vi "CreateAlertDialog.vi"(0 "reference in":refnum<class "LcWebView.lvclass">, 5 "Error In":errorcluster) -> (14 "reference out":refnum<class "LcWebView.lvclass">, 19 "Error Out":errorcluster)   [LabVIEW 2018, in "LcWebView.lvclass"]
uses:
  LcWebView.lvclass
panel:
  out "Loaded":bool
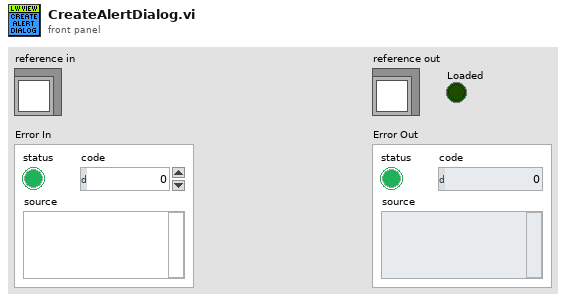
[diagram p1: front panel]
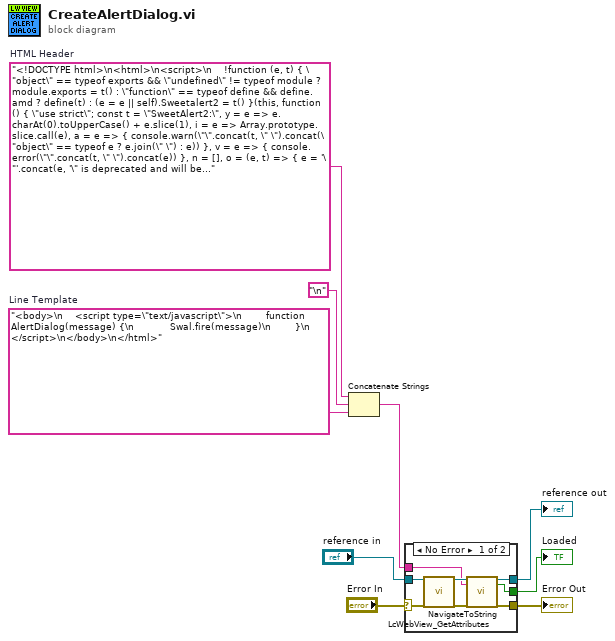
[diagram p0: block diagram]
diagram:
  w2 = "<body>\n    <script type=\"text/javascript\">\n        function AlertDialog(message) {\n            Swal.fire(message)\n        }\n    </script>\n</body>\n</html>"  # Line Template
  w4 = "<!DOCTYPE html>\n<html>\n<script>\n    !function (e, t) { \"object\" == typeof exports && \"undefined\" != typeof module ? module.exports = t() : \"function\" == typeof define && define.amd ? define(t) : (e = e || self).Sweetalert2 = t() }(this, function () { \"use strict\"; const t = \"SweetAlert2:\", y = e => e.charAt(0).toUpperCase() + e.slice(1), i = e => Array.prototype.slice.call(e), a = e => { console.warn(\"\".concat(t, \" \").concat(\"object\" == typeof e ? e.join(\" \") : e)) }, v = e => { console.error(\"\".concat(t, \" \").concat(e)) }, n = [], o = (e, t) => { e = '\"'.concat(e, '\" is deprecated and will be removed in the next major release. Please use \"').concat(t, '\" instead.'), n.includes(e) || (n.push(e), a(e)) }, w = e => \"function\" == typeof e ? e() : e, C = e => e && \"function\" == typeof e.toPromise, k = e => C(e) ? e.toPromise() : Promise.resolve(e), A = e => e && Promise.resolve(e) === e, r = { title: \"\", titleText: \"\", text: \"\", html: \"\", footer: \"\", icon: void 0, iconColor: void 0, iconHtml: void 0, template: void 0, toast: !1, showClass: { popup: \"swal2-show\", backdrop: \"swal2-backdrop-show\", icon: \"swal2-icon-show\" }, hideClass: { popup: \"swal2-hide\", backdrop: \"swal2-backdrop-hide\", icon: \"swal2-icon-hide\" }, customClass: {}, target: \"body\", color: void 0, backdrop: !0, heightAuto: !0, allowOutsideClick: !0, allowEscapeKey: !0, allowEnterKey: !0, stopKeydownPropagation: !0, keydownListenerCapture: !1, showConfirmButton: !0, showDenyButton: !1, showCancelButton: !1, preConfirm: void 0, preDeny: void 0, confirmButtonText: \"OK\", confirmButtonAriaLabel: \"\", confirmButtonColor: void 0, denyButtonText: \"No\", denyButtonAriaLabel: \"\", denyButtonColor: void 0, cancelButtonText: \"Cancel\", cancelButtonAriaLabel: \"\", cancelButtonColor: void 0, buttonsStyling: !0, reverseButtons: !1, focusConfirm: !0, focusDeny: !1, focusCancel: !1, returnFocus: !0, showCloseButton: !1, closeButtonHtml: \"&times;\", closeButtonAriaLabel: \"Close this dialog\", loaderHtml: \"\", showLoaderOnConfirm: !1, showLoaderOnDeny: !1, imageUrl: void 0, imageWidth: void 0, imageHeight: void 0, imageAlt: \"\", timer: void 0, timerProgressBar: !1, width: void 0, padding: void 0, background: void 0, input: void 0, inputPlaceholder: \"\", inputLabel: \"\", inputValue: \"\", inputOptions: {}, inputAutoTrim: !0, inputAttributes: {}, inputValidator: void 0, returnInputValueOnDeny: !1, validationMessage: void 0, grow: !1, position: \"center\", progressSteps: [], currentProgressStep: void 0, progressStepsDistance: void 0, willOpen: void 0, didOpen: void 0, didRender: void 0, willClose: void 0, didClose: void 0, didDestroy: void 0, scrollbarPadding: !0 }, s = [\"allowEscapeKey\", \"allowOutsideClick\", \"background\", \"buttonsStyling\", \"cancelButtonAriaLabel\", \"cancelButtonColor\", \"cancelButtonText\", \"closeButtonAriaLabel\", \"closeButtonHtml\", \"color\", \"confirmButtonAriaLabel\", \"confirmButtonColor\", \"confirmButtonText\", \"currentProgressStep\", \"customClass\", \"denyButtonAriaLabel\", \"denyButtonColor\", \"denyButtonText\", \"didClose\", \"didDestroy\", \"footer\", \"hideClass\", \"html\", \"icon\", \"iconColor\", \"iconHtml\", \"imageAlt\", \"imageHeight\", \"imageUrl\", \"imageWidth\", \"preConfirm\", \"preDeny\", \"progressSteps\", \"returnFocus\", \"reverseButtons\", \"showCancelButton\", \"showCloseButton\", \"showConfirmButton\", \"showDenyButton\", \"text\", \"title\", \"titleText\", \"willClose\"], c = {}, P = [\"allowOutsideClick\", \"allowEnterKey\", \"backdrop\", \"focusConfirm\", \"focusDeny\", \"focusCancel\", \"returnFocus\", \"heightAuto\", \"keydownListenerCapture\"], B = e => Object.prototype.hasOwnProperty.call(r, e), x = e => -1 !== s.indexOf(e), E = e => c[e], T = e => { !e.backdrop && e.allowOutsideClick && a('\"allowOutsideClick\" parameter requires `backdrop` parameter to be set to `true`'); for (const n in e) t = n, B(t) || a('Unknown parameter \"'.concat(t, '\"')), e.toast && (t = n, P.includes(t) && a('The parameter \"'.concat(t, '\" is incompatible with toasts'))), t = n, E(t) && o(t, E(t)); var t }; var e = e => { const t = {}; for (const n in e) t[e[n]] = \"swal2-\" + e[n]; return t }; const p = e([\"container\", \"shown\", \"height-auto\", \"iosfix\", \"popup\", \"modal\", \"no-backdrop\", \"no-transition\", \"toast\", \"toast-shown\", \"show\", \"hide\", \"close\", \"title\", \"html-container\", \"actions\", \"confirm\", \"deny\", \"cancel\", \"default-outline\", \"footer\", \"icon\", \"icon-content\", \"image\", \"input\", \"file\", \"range\", \"select\", \"radio\", \"checkbox\", \"label\", \"textarea\", \"inputerror\", \"input-label\", \"validation-message\", \"progress-steps\", \"active-progress-step\", \"progress-step\", \"progress-step-line\", \"loader\", \"loading\", \"styled\", \"top\", \"top-start\", \"top-end\", \"top-left\", \"top-right\", \"center\", \"center-start\", \"center-end\", \"center-left\", \"center-right\", \"bottom\", \"bottom-start\", \"bottom-end\", \"bottom-left\", \"bottom-right\", \"grow-row\", \"grow-column\", \"grow-fullscreen\", \"rtl\", \"timer-progress-bar\", \"timer-progress-bar-container\", \"scrollbar-measure\", \"icon-success\", \"icon-warning\", \"icon-info\", \"icon-question\", \"icon-error\"]), S = e([\"success\", \"warning\", \"info\", \"question\", \"error\"]), m = () => document.body.querySelector(\".\".concat(p.container)), L = e => { const t = m(); return t ? t.querySelector(e) : null }, O = e => L(\".\".concat(e)), g = () => O(p.popup), j = () => O(p.icon), M = () => O(p.title), D = () => O(p[\"html-container\"]), I = () => O(p.image), H = () => O(p[\"progress-steps\"]), q = () => O(p[\"validation-message\"]), V = () => L(\".\".concat(p.actions, \" .\").concat(p.confirm)), N = () => L(\".\".concat(p.actions, \" .\").concat(p.deny)); const R = () => L(\".\".concat(p.loader)), F = () => L(\".\".concat(p.actions, \" .\").concat(p.cancel)), U = () => O(p.actions), W = () => O(p.footer), z = () => O(p[\"timer-progress-bar\"]), _ = () => O(p.close), K = () => { const e = i(g().querySelectorAll('[tabindex]:not([tabindex=\"-1\"]):not([tabindex=\"0\"])')).sort((e, t) => { e = parseInt(e.getAttribute(\"tabindex\")), t = parseInt(t.getAttribute(\"tabindex\")); return t < e ? 1 : e < t ? -1 : 0 }); var t = i(g().querySelectorAll('\\n  a[href],\\n  area[href],\\n  input:not([disabled]),\\n  select:not([disabled]),\\n  textarea:not([disabled]),\\n  button:not([disabled]),\\n  iframe,\\n  object,\\n  embed,\\n  [tabindex=\"0\"],\\n  [contenteditable],\\n  audio[controls],\\n  video[controls],\\n  summary\\n')).filter(e => \"-1\" !== e.getAttribute(\"tabindex\")); return (t => { const n = []; for (let e = 0; e < t.length; e++)-1 === n.indexOf(t[e]) && n.push(t[e]); return n })(e.concat(t)).filter(e => ce(e)) }, Y = () => !$(document.body, p[\"toast-shown\"]) && !$(document.body, p[\"no-backdrop\"]), Z = () => g() && $(g(), p.toast); function J(e) { var t = 1 < arguments.length && void 0 !== arguments[1] && arguments[1]; const n = z(); ce(n) && (t && (n.style.transition = \"none\", n.style.width = \"100%\"), setTimeout(() => { n.style.transition = \"width \".concat(e / 1e3, \"s linear\"), n.style.width = \"0%\" }, 10)) } const X = { previousBodyPadding: null }, l = (t, e) => { if (t.textContent = \"\", e) { const n = new DOMParser, o = n.parseFromString(e, \"text/html\"); i(o.querySelector(\"head\").childNodes).forEach(e => { t.appendChild(e) }), i(o.querySelector(\"body\").childNodes).forEach(e => { t.appendChild(e) }) } }, $ = (t, e) => { if (!e) return !1; var n = e.split(/\\s+/); for (let e = 0; e < n.length; e++)if (!t.classList.contains(n[e])) return !1; return !0 }, G = (t, n) => { i(t.classList).forEach(e => { Object.values(p).includes(e) || Object.values(S).includes(e) || Object.values(n.showClass).includes(e) || t.classList.remove(e) }) }, Q = (e, t, n) => { if (G(e, t), t.customClass && t.customClass[n]) { if (\"string\" != typeof t.customClass[n] && !t.customClass[n].forEach) return a(\"Invalid type of customClass.\".concat(n, '! Expected string or iterable object, got \"').concat(typeof t.customClass[n], '\"')); u(e, t.customClass[n]) } }, ee = (e, t) => { if (!t) return null; switch (t) { case \"select\": case \"textarea\": case \"file\": return e.querySelector(\".\".concat(p.popup, \" > .\").concat(p[t])); case \"checkbox\": return e.querySelector(\".\".concat(p.popup, \" > .\").concat(p.checkbox, \" input\")); case \"radio\": return e.querySelector(\".\".concat(p.popup, \" > .\").concat(p.radio, \" input:checked\")) || e.querySelector(\".\".concat(p.popup, \" > .\").concat(p.radio, \" input:first-child\")); case \"range\": return e.querySelector(\".\".concat(p.popup, \" > .\").concat(p.range, \" input\")); default: return e.querySelector(\".\".concat(p.popup, \" > .\").concat(p.input)) } }, te = e => { var t; e.focus(), \"file\" !== e.type && (t = e.value, e.value = \"\", e.value = t) }, ne = (e, t, n) => { e && t && (t = \"string\" == typeof t ? t.split(/\\s+/).filter(Boolean) : t).forEach(t => { Array.isArray(e) ? e.forEach(e => { n ? e.classList.add(t) : e.classList.remove(t) }) : n ? e.classList.add(t) : e.classList.remove(t) }) }, u = (e, t) => { ne(e, t, !0) }, oe = (e, t) => { ne(e, t, !1) }, ie = (e, t) => { var n = i(e.childNodes); for (let e = 0; e < n.length; e++)if ($(n[e], t)) return n[e] }, ae = (e, t, n) => { (n = n === \"\".concat(parseInt(n)) ? parseInt(n) : n) || 0 === parseInt(n) ? e.style[t] = \"number\" == typeof n ? \"\".concat(n, \"px\") : n : e.style.removeProperty(t) }, d = function (e) { e.style.display = 1 < arguments.length && void 0 !== arguments[1] ? arguments[1] : \"flex\" }, h = e => { e.style.display = \"none\" }, re = (e, t, n, o) => { const i = e.querySelector(t); i && (i.style[n] = o) }, se = (e, t, n) => { t ? d(e, n) : h(e) }, ce = e => !(!e || !(e.offsetWidth || e.offsetHeight || e.getClientRects().length)), le = () => !ce(V()) && !ce(N()) && !ce(F()), ue = e => !!(e.scrollHeight > e.clientHeight), de = e => { const t = window.getComputedStyle(e); var e = parseFloat(t.getPropertyValue(\"animation-duration\") || \"0\"), n = parseFloat(t.getPropertyValue(\"transition-duration\") || \"0\"); return 0 < e || 0 < n }, pe = () => \"undefined\" == typeof window || \"undefined\" == typeof document, me = 100, f = {}, ge = () => { f.previousActiveElement && f.previousActiveElement.focus ? (f.previousActiveElement.focus(), f.previousActiveElement = null) : document.body && document.body.focus() }, he = o => new Promise(e => { if (!o) return e(); var t = window.scrollX, n = window.scrollY; f.restoreFocusTimeout = setTimeout(() => { ge(), e() }, me), window.scrollTo(t, n) }), fe = '\\n <div aria-labelledby=\"'.concat(p.title, '\" aria-describedby=\"').concat(p[\"html-container\"], '\" class=\"').concat(p.popup, '\" tabindex=\"-1\">\\n   <button type=\"button\" class=\"').concat(p.close, '\"></button>\\n   <ul class=\"').concat(p[\"progress-steps\"], '\"></ul>\\n   <div class=\"').concat(p.icon, '\"></div>\\n   <img class=\"').concat(p.image, '\" />\\n   <h2 class=\"').concat(p.title, '\" id=\"').concat(p.title, '\"></h2>\\n   <div class=\"').concat(p[\"html-container\"], '\" id=\"').concat(p[\"html-container\"], '\"></div>\\n   <input class=\"').concat(p.input, '\" />\\n   <input type=\"file\" class=\"').concat(p.file, '\" />\\n   <div class=\"').concat(p.range, '\">\\n     <input type=\"range\" />\\n     <output></output>\\n   </div>\\n   <select class=\"').concat(p.select, '\"></select>\\n   <div class=\"').concat(p.radio, '\"></div>\\n   <label for=\"').concat(p.checkbox, '\" class=\"').concat(p.checkbox, '\">\\n     <input type=\"checkbox\" />\\n     <span class=\"').concat(p.label, '\"></span>\\n   </label>\\n   <textarea class=\"').concat(p.textarea, '\"></textarea>\\n   <div class=\"').concat(p[\"validation-message\"], '\" id=\"').concat(p[\"validation-message\"], '\"></div>\\n   <div class=\"').concat(p.actions, '\">\\n     <div class=\"').concat(p.loader, '\"></div>\\n     <button type=\"button\" class=\"').concat(p.confirm, '\"></button>\\n     <button type=\"button\" class=\"').concat(p.deny, '\"></button>\\n     <button type=\"button\" class=\"').concat(p.cancel, '\"></button>\\n   </div>\\n   <div class=\"').concat(p.footer, '\"></div>\\n   <div class=\"').concat(p[\"timer-progress-bar-container\"], '\">\\n     <div class=\"').concat(p[\"timer-progress-bar\"], '\"></div>\\n   </div>\\n </div>\\n').replace(/(^|\\n)\\s*/g, \"\"), be = () => { const e = m(); return !!e && (e.remove(), oe([document.documentElement, document.body], [p[\"no-backdrop\"], p[\"toast-shown\"], p[\"has-column\"]]), !0) }, ye = () => { f.currentInstance.resetValidationMessage() }, ve = () => { const e = g(), t = ie(e, p.input), n = ie(e, p.file), o = e.querySelector(\".\".concat(p.range, \" input\")), i = e.querySelector(\".\".concat(p.range, \" output\")), a = ie(e, p.select), r = e.querySelector(\".\".concat(p.checkbox, \" input\")), s = ie(e, p.textarea); t.oninput = ye, n.onchange = ye, a.onchange = ye, r.onchange = ye, s.oninput = ye, o.oninput = () => { ye(), i.value = o.value }, o.onchange = () => { ye(), o.nextSibling.value = o.value } }, we = e => \"string\" == typeof e ? document.querySelector(e) : e, Ce = e => { const t = g(); t.setAttribute(\"role\", e.toast ? \"alert\" : \"dialog\"), t.setAttribute(\"aria-live\", e.toast ? \"polite\" : \"assertive\"), e.toast || t.setAttribute(\"aria-modal\", \"true\") }, ke = e => { \"rtl\" === window.getComputedStyle(e).direction && u(m(), p.rtl) }, Ae = (e, t) => { if (e instanceof HTMLElement) t.appendChild(e); else if (\"object\" == typeof e) { var n = e, o = t; if (n.jquery) Pe(o, n); else l(o, n.toString()) } else e && l(t, e) }, Pe = (t, n) => { if (t.textContent = \"\", 0 in n) for (let e = 0; e in n; e++)t.appendChild(n[e].cloneNode(!0)); else t.appendChild(n.cloneNode(!0)) }, Be = (() => { if (pe()) return !1; var e = document.createElement(\"div\"), t = { WebkitAnimation: \"webkitAnimationEnd\", animation: \"animationend\" }; for (const n in t) if (Object.prototype.hasOwnProperty.call(t, n) && void 0 !== e.style[n]) return t[n]; return !1 })(), xe = (e, t) => { var n, o, i, a, r, s = U(), c = R(); (t.showConfirmButton || t.showDenyButton || t.showCancelButton ? d : h)(s), Q(s, t, \"actions\"), s = s, n = c, o = t, i = V(), a = N(), r = F(), Ee(i, \"confirm\", o), Ee(a, \"deny\", o), Ee(r, \"cancel\", o), function (e, t, n, o) { if (!o.buttonsStyling) return oe([e, t, n], p.styled); u([e, t, n], p.styled), o.confirmButtonColor && (e.style.backgroundColor = o.confirmButtonColor, u(e, p[\"default-outline\"])); o.denyButtonColor && (t.style.backgroundColor = o.denyButtonColor, u(t, p[\"default-outline\"])); o.cancelButtonColor && (n.style.backgroundColor = o.cancelButtonColor, u(n, p[\"default-outline\"])) }(i, a, r, o), o.reverseButtons && (o.toast ? (s.insertBefore(r, i), s.insertBefore(a, i)) : (s.insertBefore(r, n), s.insertBefore(a, n), s.insertBefore(i, n))), l(c, t.loaderHtml), Q(c, t, \"loader\") }; function Ee(e, t, n) { se(e, n[\"show\".concat(y(t), \"Button\")], \"inline-block\"), l(e, n[\"\".concat(t, \"ButtonText\")]), e.setAttribute(\"aria-label\", n[\"\".concat(t, \"ButtonAriaLabel\")]), e.className = p[t], Q(e, n, \"\".concat(t, \"Button\")), u(e, n[\"\".concat(t, \"ButtonClass\")]) } const Te = (e, t) => { var n, o, i = m(); i && (o = i, \"string\" == typeof (n = t.backdrop) ? o.style.background = n : n || u([document.documentElement, document.body], p[\"no-backdrop\"]), o = i, (n = t.position) in p ? u(o, p[n]) : (a('The \"position\" parameter is not valid, defaulting to \"center\"'), u(o, p.center)), n = i, !(o = t.grow) || \"string\" != typeof o || (o = \"grow-\".concat(o)) in p && u(n, p[o]), Q(i, t, \"container\")) }; var b = { awaitingPromise: new WeakMap, promise: new WeakMap, innerParams: new WeakMap, domCache: new WeakMap }; const Se = [\"input\", \"file\", \"range\", \"select\", \"radio\", \"checkbox\", \"textarea\"], Le = (e, r) => { const s = g(); var t, e = b.innerParams.get(e); const c = !e || r.input !== e.input; Se.forEach(e => { var t = p[e]; const n = ie(s, t); { var o = r.inputAttributes; const i = ee(g(), e); if (i) { Oe(i); for (const a in o) i.setAttribute(a, o[a]) } } n.className = t, c && h(n) }), r.input && (c && (e => { if (!Ie[e.input]) return v('Unexpected type of input! Expected \"text\", \"email\", \"password\", \"number\", \"tel\", \"select\", \"radio\", \"checkbox\", \"textarea\", \"file\" or \"url\", got \"'.concat(e.input, '\"')); const t = De(e.input), n = Ie[e.input](t, e); d(n), setTimeout(() => { te(n) }) })(r), e = r, t = De(e.input), e.customClass && u(t, e.customClass.input)) }, Oe = t => { for (let e = 0; e < t.attributes.length; e++) { var n = t.attributes[e].name;[\"type\", \"value\", \"style\"].includes(n) || t.removeAttribute(n) } }, je = (e, t) => { e.placeholder && !t.inputPlaceholder || (e.placeholder = t.inputPlaceholder) }, Me = (e, t, n) => { if (n.inputLabel) { e.id = p.input; const i = document.createElement(\"label\"); var o = p[\"input-label\"]; i.setAttribute(\"for\", e.id), i.className = o, u(i, n.customClass.inputLabel), i.innerText = n.inputLabel, t.insertAdjacentElement(\"beforebegin\", i) } }, De = e => { e = p[e] || p.input; return ie(g(), e) }, Ie = {}, He = (Ie.text = Ie.email = Ie.password = Ie.number = Ie.tel = Ie.url = (e, t) => (\"string\" == typeof t.inputValue || \"number\" == typeof t.inputValue ? e.value = t.inputValue : A(t.inputValue) || a('Unexpected type of inputValue! Expected \"string\", \"number\" or \"Promise\", got \"'.concat(typeof t.inputValue, '\"')), Me(e, e, t), je(e, t), e.type = t.input, e), Ie.file = (e, t) => (Me(e, e, t), je(e, t), e), Ie.range = (e, t) => { const n = e.querySelector(\"input\"), o = e.querySelector(\"output\"); return n.value = t.inputValue, n.type = t.input, o.value = t.inputValue, Me(n, e, t), e }, Ie.select = (e, t) => { if (e.textContent = \"\", t.inputPlaceholder) { const n = document.createElement(\"option\"); l(n, t.inputPlaceholder), n.value = \"\", n.disabled = !0, n.selected = !0, e.appendChild(n) } return Me(e, e, t), e }, Ie.radio = e => (e.textContent = \"\", e), Ie.checkbox = (e, t) => { const n = ee(g(), \"checkbox\"); n.value = \"1\", n.id = p.checkbox, n.checked = Boolean(t.inputValue); var o = e.querySelector(\"span\"); return l(o, t.inputPlaceholder), e }, Ie.textarea = (n, e) => { n.value = e.inputValue, je(n, e), Me(n, n, e); return setTimeout(() => { if (\"MutationObserver\" in window) { const t = parseInt(window.getComputedStyle(g()).width); new MutationObserver(() => { var e = n.offsetWidth + (e = n, parseInt(window.getComputedStyle(e).marginLeft) + parseInt(window.getComputedStyle(e).marginRight)); e > t ? g().style.width = \"\".concat(e, \"px\") : g().style.width = null }).observe(n, { attributes: !0, attributeFilter: [\"style\"] }) } }), n }, (e, t) => { const n = D(); Q(n, t, \"htmlContainer\"), t.html ? (Ae(t.html, n), d(n, \"block\")) : t.text ? (n.textContent = t.text, d(n, \"block\")) : h(n), Le(e, t) }), qe = (e, t) => { var n = W(); se(n, t.footer), t.footer && Ae(t.footer, n), Q(n, t, \"footer\") }, Ve = (e, t) => { const n = _(); l(n, t.closeButtonHtml), Q(n, t, \"closeButton\"), se(n, t.showCloseButton), n.setAttribute(\"aria-label\", t.closeButtonAriaLabel) }, Ne = (e, t) => { var e = b.innerParams.get(e), n = j(); return e && t.icon === e.icon ? (ze(n, t), void Re(n, t)) : t.icon || t.iconHtml ? t.icon && -1 === Object.keys(S).indexOf(t.icon) ? (v('Unknown icon! Expected \"success\", \"error\", \"warning\", \"info\" or \"question\", got \"'.concat(t.icon, '\"')), h(n)) : (d(n), ze(n, t), Re(n, t), void u(n, t.showClass.icon)) : h(n) }, Re = (e, t) => { for (const n in S) t.icon !== n && oe(e, S[n]); u(e, S[t.icon]), _e(e, t), Fe(), Q(e, t, \"icon\") }, Fe = () => { const e = g(); var t = window.getComputedStyle(e).getPropertyValue(\"background-color\"); const n = e.querySelectorAll(\"[class^=swal2-success-circular-line], .swal2-success-fix\"); for (let e = 0; e < n.length; e++)n[e].style.backgroundColor = t }, Ue = '\\n  <div class=\"swal2-success-circular-line-left\"></div>\\n  <span class=\"swal2-success-line-tip\"></span> <span class=\"swal2-success-line-long\"></span>\\n  <div class=\"swal2-success-ring\"></div> <div class=\"swal2-success-fix\"></div>\\n  <div class=\"swal2-success-circular-line-right\"></div>\\n', We = '\\n  <span class=\"swal2-x-mark\">\\n    <span class=\"swal2-x-mark-line-left\"></span>\\n    <span class=\"swal2-x-mark-line-right\"></span>\\n  </span>\\n', ze = (e, t) => { var n; e.textContent = \"\", t.iconHtml ? l(e, Ke(t.iconHtml)) : \"success\" === t.icon ? l(e, Ue) : \"error\" === t.icon ? l(e, We) : (n = { question: \"?\", warning: \"!\", info: \"i\" }, l(e, Ke(n[t.icon]))) }, _e = (e, t) => { if (t.iconColor) { e.style.color = t.iconColor, e.style.borderColor = t.iconColor; for (const n of [\".swal2-success-line-tip\", \".swal2-success-line-long\", \".swal2-x-mark-line-left\", \".swal2-x-mark-line-right\"]) re(e, n, \"backgroundColor\", t.iconColor); re(e, \".swal2-success-ring\", \"borderColor\", t.iconColor) } }, Ke = e => '<div class=\"'.concat(p[\"icon-content\"], '\">').concat(e, \"</div>\"), Ye = (e, t) => { const n = I(); if (!t.imageUrl) return h(n); d(n, \"\"), n.setAttribute(\"src\", t.imageUrl), n.setAttribute(\"alt\", t.imageAlt), ae(n, \"width\", t.imageWidth), ae(n, \"height\", t.imageHeight), n.className = p.image, Q(n, t, \"image\") }, Ze = (e, o) => { const i = H(); if (!o.progressSteps || 0 === o.progressSteps.length) return h(i); d(i), i.textContent = \"\", o.currentProgressStep >= o.progressSteps.length && a(\"Invalid currentProgressStep parameter, it should be less than progressSteps.length (currentProgressStep like JS arrays starts from 0)\"), o.progressSteps.forEach((e, t) => { e = e, n = document.createElement(\"li\"), u(n, p[\"progress-step\"]), l(n, e); var n, e = n; i.appendChild(e), t === o.currentProgressStep && u(e, p[\"active-progress-step\"]), t !== o.progressSteps.length - 1 && (n = (e => { const t = document.createElement(\"li\"); return u(t, p[\"progress-step-line\"]), e.progressStepsDistance && (t.style.width = e.progressStepsDistance), t })(o), i.appendChild(n)) }) }, Je = (e, t) => { const n = M(); se(n, t.title || t.titleText, \"block\"), t.title && Ae(t.title, n), t.titleText && (n.innerText = t.titleText), Q(n, t, \"title\") }, Xe = (e, t) => { var n = m(); const o = g(); t.toast ? (ae(n, \"width\", t.width), o.style.width = \"100%\", o.insertBefore(R(), j())) : ae(o, \"width\", t.width), ae(o, \"padding\", t.padding), t.color && (o.style.color = t.color), t.background && (o.style.background = t.background), h(q()); n = o; (n.className = \"\".concat(p.popup, \" \").concat(ce(n) ? t.showClass.popup : \"\"), t.toast) ? (u([document.documentElement, document.body], p[\"toast-shown\"]), u(n, p.toast)) : u(n, p.modal); Q(n, t, \"popup\"), \"string\" == typeof t.customClass && u(n, t.customClass); t.icon && u(n, p[\"icon-\".concat(t.icon)]) }, $e = (e, t) => { Xe(e, t), Te(e, t), Ze(e, t), Ne(e, t), Ye(e, t), Je(e, t), Ve(e, t), He(e, t), xe(e, t), qe(e, t), \"function\" == typeof t.didRender && t.didRender(g()) }, Ge = Object.freeze({ cancel: \"cancel\", backdrop: \"backdrop\", close: \"close\", esc: \"esc\", timer: \"timer\" }), Qe = () => { const e = i(document.body.children); e.forEach(e => { e === m() || e.contains(m()) || (e.hasAttribute(\"aria-hidden\") && e.setAttribute(\"data-previous-aria-hidden\", e.getAttribute(\"aria-hidden\")), e.setAttribute(\"aria-hidden\", \"true\")) }) }, et = () => { const e = i(document.body.children); e.forEach(e => { e.hasAttribute(\"data-previous-aria-hidden\") ? (e.setAttribute(\"aria-hidden\", e.getAttribute(\"data-previous-aria-hidden\")), e.removeAttribute(\"data-previous-aria-hidden\")) : e.removeAttribute(\"aria-hidden\") }) }, tt = [\"swal-title\", \"swal-html\", \"swal-footer\"], nt = e => { const n = {}; return i(e.querySelectorAll(\"swal-param\")).forEach(e => { lt(e, [\"name\", \"value\"]); var t = e.getAttribute(\"name\"), e = e.getAttribute(\"value\"); \"boolean\" == typeof r[t] && \"false\" === e && (n[t] = !1), \"object\" == typeof r[t] && (n[t] = JSON.parse(e)) }), n }, ot = e => { const n = {}; return i(e.querySelectorAll(\"swal-button\")).forEach(e => { lt(e, [\"type\", \"color\", \"aria-label\"]); var t = e.getAttribute(\"type\"); n[\"\".concat(t, \"ButtonText\")] = e.innerHTML, n[\"show\".concat(y(t), \"Button\")] = !0, e.hasAttribute(\"color\") && (n[\"\".concat(t, \"ButtonColor\")] = e.getAttribute(\"color\")), e.hasAttribute(\"aria-label\") && (n[\"\".concat(t, \"ButtonAriaLabel\")] = e.getAttribute(\"aria-label\")) }), n }, it = e => { const t = {}, n = e.querySelector(\"swal-image\"); return n && (lt(n, [\"src\", \"width\", \"height\", \"alt\"]), n.hasAttribute(\"src\") && (t.imageUrl = n.getAttribute(\"src\")), n.hasAttribute(\"width\") && (t.imageWidth = n.getAttribute(\"width\")), n.hasAttribute(\"height\") && (t.imageHeight = n.getAttribute(\"height\")), n.hasAttribute(\"alt\") && (t.imageAlt = n.getAttribute(\"alt\"))), t }, at = e => { const t = {}, n = e.querySelector(\"swal-icon\"); return n && (lt(n, [\"type\", \"color\"]), n.hasAttribute(\"type\") && (t.icon = n.getAttribute(\"type\")), n.hasAttribute(\"color\") && (t.iconColor = n.getAttribute(\"color\")), t.iconHtml = n.innerHTML), t }, rt = e => { const n = {}, t = e.querySelector(\"swal-input\"); t && (lt(t, [\"type\", \"label\", \"placeholder\", \"value\"]), n.input = t.getAttribute(\"type\") || \"text\", t.hasAttribute(\"label\") && (n.inputLabel = t.getAttribute(\"label\")), t.hasAttribute(\"placeholder\") && (n.inputPlaceholder = t.getAttribute(\"placeholder\")), t.hasAttribute(\"value\") && (n.inputValue = t.getAttribute(\"value\"))); e = e.querySelectorAll(\"swal-input-option\"); return e.length && (n.inputOptions = {}, i(e).forEach(e => { lt(e, [\"value\"]); var t = e.getAttribute(\"value\"), e = e.innerHTML; n.inputOptions[t] = e })), n }, st = (e, t) => { const n = {}; for (const o in t) { const i = t[o], a = e.querySelector(i); a && (lt(a, []), n[i.replace(/^swal-/, \"\")] = a.innerHTML.trim()) } return n }, ct = e => { const t = tt.concat([\"swal-param\", \"swal-button\", \"swal-image\", \"swal-icon\", \"swal-input\", \"swal-input-option\"]); i(e.children).forEach(e => { e = e.tagName.toLowerCase(); -1 === t.indexOf(e) && a(\"Unrecognized element <\".concat(e, \">\")) }) }, lt = (t, n) => { i(t.attributes).forEach(e => { -1 === n.indexOf(e.name) && a(['Unrecognized attribute \"'.concat(e.name, '\" on <').concat(t.tagName.toLowerCase(), \">.\"), \"\".concat(n.length ? \"Allowed attributes are: \".concat(n.join(\", \")) : \"To set the value, use HTML within the element.\")]) }) }; var ut = { email: (e, t) => /^[a-zA-Z0-9.+_-]+@[a-zA-Z0-9.-]+\\.[a-zA-Z0-9-]{2,24}$/.test(e) ? Promise.resolve() : Promise.resolve(t || \"Invalid email address\"), url: (e, t) => /^https?:\\/\\/(www\\.)?[-a-zA-Z0-9@:%._+~#=]{1,256}\\.[a-z]{2,63}\\b([-a-zA-Z0-9@:%_+.~#?&/=]*)$/.test(e) ? Promise.resolve() : Promise.resolve(t || \"Invalid URL\") }; function dt(e) { (t = e).inputValidator || Object.keys(ut).forEach(e => { t.input === e && (t.inputValidator = ut[e]) }), e.showLoaderOnConfirm && !e.preConfirm && a(\"showLoaderOnConfirm is set to true, but preConfirm is not defined.\\nshowLoaderOnConfirm should be used together with preConfirm, see usage example:\\nhttps://sweetalert2.github.io/#ajax-request\"), (n = e).target && (\"string\" != typeof n.target || document.querySelector(n.target)) && (\"string\" == typeof n.target || n.target.appendChild) || (a('Target parameter is not valid, defaulting to \"body\"'), n.target = \"body\"), \"string\" == typeof e.title && (e.title = e.title.split(\"\\n\").join(\"<br />\")); var t, n = e, e = be(); if (pe()) v(\"SweetAlert2 requires document to initialize\"); else { const o = document.createElement(\"div\"), i = (o.className = p.container, e && u(o, p[\"no-transition\"]), l(o, fe), we(n.target)); i.appendChild(o), Ce(n), ke(i), ve() } } class pt { constructor(e, t) { this.callback = e, this.remaining = t, this.running = !1, this.start() } start() { return this.running || (this.running = !0, this.started = new Date, this.id = setTimeout(this.callback, this.remaining)), this.remaining } stop() { return this.running && (this.running = !1, clearTimeout(this.id), this.remaining -= (new Date).getTime() - this.started.getTime()), this.remaining } increase(e) { var t = this.running; return t && this.stop(), this.remaining += e, t && this.start(), this.remaining } getTimerLeft() { return this.running && (this.stop(), this.start()), this.remaining } isRunning() { return this.running } } const mt = () => { null === X.previousBodyPadding && document.body.scrollHeight > window.innerHeight && (X.previousBodyPadding = parseInt(window.getComputedStyle(document.body).getPropertyValue(\"padding-right\")), document.body.style.paddingRight = \"\".concat(X.previousBodyPadding + (() => { const e = document.createElement(\"div\"); e.className = p[\"scrollbar-measure\"], document.body.appendChild(e); var t = e.getBoundingClientRect().width - e.clientWidth; return document.body.removeChild(e), t })(), \"px\")) }, gt = () => { null !== X.previousBodyPadding && (document.body.style.paddingRight = \"\".concat(X.previousBodyPadding, \"px\"), X.previousBodyPadding = null) }, ht = () => { var e = /iPad|iPhone|iPod/.test(navigator.userAgent) && !window.MSStream || \"MacIntel\" === navigator.platform && 1 < navigator.maxTouchPoints; if (e && !$(document.body, p.iosfix)) { var t, e = document.body.scrollTop; document.body.style.top = \"\".concat(-1 * e, \"px\"), u(document.body, p.iosfix); { const n = m(); let t; n.ontouchstart = e => { t = ft(e) }, n.ontouchmove = e => { t && (e.preventDefault(), e.stopPropagation()) } } { const o = navigator.userAgent, i = !!o.match(/iPad/i) || !!o.match(/iPhone/i), a = !!o.match(/WebKit/i), r = i && a && !o.match(/CriOS/i); r && (t = 44, g().scrollHeight > window.innerHeight - 44 && (m().style.paddingBottom = \"\".concat(44, \"px\"))) } } }, ft = e => { var t, n = e.target, o = m(); return !((t = e).touches && t.touches.length && \"stylus\" === t.touches[0].touchType || (t = e).touches && 1 < t.touches.length) && (n === o || !(ue(o) || \"INPUT\" === n.tagName || \"TEXTAREA\" === n.tagName || ue(D()) && D().contains(n))) }, bt = () => { var e; $(document.body, p.iosfix) && (e = parseInt(document.body.style.top, 10), oe(document.body, p.iosfix), document.body.style.top = \"\", document.body.scrollTop = -1 * e) }, yt = 10, vt = e => { const t = g(); if (e.target === t) { const n = m(); t.removeEventListener(Be, vt), n.style.overflowY = \"auto\" } }, wt = (e, t) => { Be && de(t) ? (e.style.overflowY = \"hidden\", t.addEventListener(Be, vt)) : e.style.overflowY = \"auto\" }, Ct = (e, t, n) => { ht(), t && \"hidden\" !== n && mt(), setTimeout(() => { e.scrollTop = 0 }) }, kt = (e, t, n) => { u(e, n.showClass.backdrop), t.style.setProperty(\"opacity\", \"0\", \"important\"), d(t, \"grid\"), setTimeout(() => { u(t, n.showClass.popup), t.style.removeProperty(\"opacity\") }, yt), u([document.documentElement, document.body], p.shown), n.heightAuto && n.backdrop && !n.toast && u([document.documentElement, document.body], p[\"height-auto\"]) }, At = e => { let t = g(); t || new vn, t = g(); var n = R(); if (Z()) h(j()); else { var o = t; const i = U(), a = R(); !e && ce(V()) && (e = V()); d(i), e && (h(e), a.setAttribute(\"data-button-to-replace\", e.className)); a.parentNode.insertBefore(a, e), u([o, i], p.loading) } d(n), t.setAttribute(\"data-loading\", !0), t.setAttribute(\"aria-busy\", !0), t.focus() }, Pt = (t, n) => { const o = g(), i = e => xt[n.input](o, Et(e), n); C(n.inputOptions) || A(n.inputOptions) ? (At(V()), k(n.inputOptions).then(e => { t.hideLoading(), i(e) })) : \"object\" == typeof n.inputOptions ? i(n.inputOptions) : v(\"Unexpected type of inputOptions! Expected object, Map or Promise, got \".concat(typeof n.inputOptions)) }, Bt = (t, n) => { const o = t.getInput(); h(o), k(n.inputValue).then(e => { o.value = \"number\" === n.input ? parseFloat(e) || 0 : \"\".concat(e), d(o), o.focus(), t.hideLoading() }).catch(e => { v(\"Error in inputValue promise: \".concat(e)), o.value = \"\", d(o), o.focus(), t.hideLoading() }) }, xt = { select: (e, t, i) => { const a = ie(e, p.select), r = (e, t, n) => { const o = document.createElement(\"option\"); o.value = n, l(o, t), o.selected = Tt(n, i.inputValue), e.appendChild(o) }; t.forEach(e => { var t = e[0]; const n = e[1]; if (Array.isArray(n)) { const o = document.createElement(\"optgroup\"); o.label = t, o.disabled = !1, a.appendChild(o), n.forEach(e => r(o, e[1], e[0])) } else r(a, n, t) }), a.focus() }, radio: (e, t, a) => { const r = ie(e, p.radio), n = (t.forEach(e => { var t = e[0], e = e[1]; const n = document.createElement(\"input\"), o = document.createElement(\"label\"), i = (n.type = \"radio\", n.name = p.radio, n.value = t, Tt(t, a.inputValue) && (n.checked = !0), document.createElement(\"span\")); l(i, e), i.className = p.label, o.appendChild(n), o.appendChild(i), r.appendChild(o) }), r.querySelectorAll(\"input\")); n.length && n[0].focus() } }, Et = n => { const o = []; return \"undefined\" != typeof Map && n instanceof Map ? n.forEach((e, t) => { let n = e; \"object\" == typeof n && (n = Et(n)), o.push([t, n]) }) : Object.keys(n).forEach(e => { let t = n[e]; \"object\" == typeof t && (t = Et(t)), o.push([e, t]) }), o }, Tt = (e, t) => t && t.toString() === e.toString(), St = (e, t) => { var n = b.innerParams.get(e); if (!n.input) return v('The \"input\" parameter is needed to be set when using returnInputValueOn'.concat(y(t))); var o = ((e, t) => { const n = e.getInput(); if (!n) return null; switch (t.input) { case \"checkbox\": return n.checked ? 1 : 0; case \"radio\": return (o = n).checked ? o.value : null; case \"file\": return (o = n).files.length ? null !== o.getAttribute(\"multiple\") ? o.files : o.files[0] : null; default: return t.inputAutoTrim ? n.value.trim() : n.value }var o })(e, n); if (n.inputValidator) { var i = e; var a = o; var r = t; const s = b.innerParams.get(i), c = (i.disableInput(), Promise.resolve().then(() => k(s.inputValidator(a, s.validationMessage)))); c.then(e => { i.enableButtons(), i.enableInput(), e ? i.showValidationMessage(e) : (\"deny\" === r ? Lt : Mt)(i, a) }) } else e.getInput().checkValidity() ? (\"deny\" === t ? Lt : Mt)(e, o) : (e.enableButtons(), e.showValidationMessage(n.validationMessage)) }, Lt = (t, n) => { const e = b.innerParams.get(t || void 0); if (e.showLoaderOnDeny && At(N()), e.preDeny) { b.awaitingPromise.set(t || void 0, !0); const o = Promise.resolve().then(() => k(e.preDeny(n, e.validationMessage))); o.then(e => { !1 === e ? t.hideLoading() : t.closePopup({ isDenied: !0, value: void 0 === e ? n : e }) }).catch(e => jt(t || void 0, e)) } else t.closePopup({ isDenied: !0, value: n }) }, Ot = (e, t) => { e.closePopup({ isConfirmed: !0, value: t }) }, jt = (e, t) => { e.rejectPromise(t) }, Mt = (t, n) => { const e = b.innerParams.get(t || void 0); if (e.showLoaderOnConfirm && At(), e.preConfirm) { t.resetValidationMessage(), b.awaitingPromise.set(t || void 0, !0); const o = Promise.resolve().then(() => k(e.preConfirm(n, e.validationMessage))); o.then(e => { ce(q()) || !1 === e ? t.hideLoading() : Ot(t, void 0 === e ? n : e) }).catch(e => jt(t || void 0, e)) } else Ot(t, n) }, Dt = (n, e, o) => { e.popup.onclick = () => { var e, t = b.innerParams.get(n); t && ((e = t).showConfirmButton || e.showDenyButton || e.showCancelButton || e.showCloseButton || t.timer || t.input) || o(Ge.close) } }; let It = !1; const Ht = t => { t.popup.onmousedown = () => { t.container.onmouseup = function (e) { t.container.onmouseup = void 0, e.target === t.container && (It = !0) } } }, qt = t => { t.container.onmousedown = () => { t.popup.onmouseup = function (e) { t.popup.onmouseup = void 0, e.target !== t.popup && !t.popup.contains(e.target) || (It = !0) } } }, Vt = (n, o, i) => { o.container.onclick = e => { var t = b.innerParams.get(n); It ? It = !1 : e.target === o.container && w(t.allowOutsideClick) && i(Ge.backdrop) } }; const Nt = () => V() && V().click(); const Rt = (e, t, n) => { const o = K(); if (o.length) return (t += n) === o.length ? t = 0 : -1 === t && (t = o.length - 1), o[t].focus(); g().focus() }, Ft = [\"ArrowRight\", \"ArrowDown\"], Ut = [\"ArrowLeft\", \"ArrowUp\"], Wt = (e, n, o) => { var i = b.innerParams.get(e); if (i) if (i.stopKeydownPropagation && n.stopPropagation(), \"Enter\" === n.key) e = e, a = n, t = i, w(t.allowEnterKey) && !a.isComposing && a.target && e.getInput() && a.target.outerHTML === e.getInput().outerHTML && ([\"textarea\", \"file\"].includes(t.input) || (Nt(), a.preventDefault())); else if (\"Tab\" !== n.key) { if ([...Ft, ...Ut].includes(n.key)) { e = n.key; const s = V(), c = N(), d = F(); if ([s, c, d].includes(document.activeElement)) { var t = Ft.includes(e) ? \"nextElementSibling\" : \"previousElementSibling\"; const l = document.activeElement[t]; l instanceof HTMLElement && l.focus() } } else if (\"Escape\" === n.key) { var a = n, e = i; if (w(e.allowEscapeKey)) { a.preventDefault(); o(Ge.esc) } } } else { e = n; o = i; var u = e.target, r = K(); let t = -1; for (let e = 0; e < r.length; e++)if (u === r[e]) { t = e; break } e.shiftKey ? Rt(o, t, -1) : Rt(o, t, 1); e.stopPropagation(), e.preventDefault() } }, zt = e => \"object\" == typeof e && e.jquery, _t = e => e instanceof Element || zt(e); const Kt = () => { if (f.timeout) { { const n = z(); var e = parseInt(window.getComputedStyle(n).width), t = (n.style.removeProperty(\"transition\"), n.style.width = \"100%\", parseInt(window.getComputedStyle(n).width)), e = e / t * 100; n.style.removeProperty(\"transition\"), n.style.width = \"\".concat(e, \"%\") } return f.timeout.stop() } }, Yt = () => { var e; if (f.timeout) return e = f.timeout.start(), J(e), e }; let Zt = !1; const Jt = {}; const Xt = t => { for (let e = t.target; e && e !== document; e = e.parentNode)for (const o in Jt) { var n = e.getAttribute(o); if (n) return void Jt[o].fire({ template: n }) } }; e = Object.freeze({ isValidParameter: B, isUpdatableParameter: x, isDeprecatedParameter: E, argsToParams: n => { const o = {}; return \"object\" != typeof n[0] || _t(n[0]) ? [\"title\", \"html\", \"icon\"].forEach((e, t) => { t = n[t]; \"string\" == typeof t || _t(t) ? o[e] = t : void 0 !== t && v(\"Unexpected type of \".concat(e, '! Expected \"string\" or \"Element\", got ').concat(typeof t)) }) : Object.assign(o, n[0]), o }, isVisible: () => ce(g()), clickConfirm: Nt, clickDeny: () => N() && N().click(), clickCancel: () => F() && F().click(), getContainer: m, getPopup: g, getTitle: M, getHtmlContainer: D, getImage: I, getIcon: j, getInputLabel: () => O(p[\"input-label\"]), getCloseButton: _, getActions: U, getConfirmButton: V, getDenyButton: N, getCancelButton: F, getLoader: R, getFooter: W, getTimerProgressBar: z, getFocusableElements: K, getValidationMessage: q, isLoading: () => g().hasAttribute(\"data-loading\"), fire: function () { for (var e = arguments.length, t = new Array(e), n = 0; n < e; n++)t[n] = arguments[n]; return new this(...t) }, mixin: function (n) { class e extends this{ _main(e, t) { return super._main(e, Object.assign({}, n, t)) } } return e }, showLoading: At, enableLoading: At, getTimerLeft: () => f.timeout && f.timeout.getTimerLeft(), stopTimer: Kt, resumeTimer: Yt, toggleTimer: () => { var e = f.timeout; return e && (e.running ? Kt : Yt)() }, increaseTimer: e => { if (f.timeout) return e = f.timeout.increase(e), J(e, !0), e }, isTimerRunning: () => f.timeout && f.timeout.isRunning(), bindClickHandler: function () { var e = 0 < arguments.length && void 0 !== arguments[0] ? arguments[0] : \"data-swal-template\"; Jt[e] = this, Zt || (document.body.addEventListener(\"click\", Xt), Zt = !0) } }); function $t() { var e, t = b.innerParams.get(this); if (t) { const n = b.domCache.get(this); h(n.loader), Z() ? t.icon && d(j()) : (t = n, (e = t.popup.getElementsByClassName(t.loader.getAttribute(\"data-button-to-replace\"))).length ? d(e[0], \"inline-block\") : le() && h(t.actions)), oe([n.popup, n.actions], p.loading), n.popup.removeAttribute(\"aria-busy\"), n.popup.removeAttribute(\"data-loading\"), n.confirmButton.disabled = !1, n.denyButton.disabled = !1, n.cancelButton.disabled = !1 } } var Gt = { swalPromiseResolve: new WeakMap, swalPromiseReject: new WeakMap }; function Qt(e, t, n, o) { Z() ? on(e, o) : (he(n).then(() => on(e, o)), f.keydownTarget.removeEventListener(\"keydown\", f.keydownHandler, { capture: f.keydownListenerCapture }), f.keydownHandlerAdded = !1), /^((?!chrome|android).)*safari/i.test(navigator.userAgent) ? (t.setAttribute(\"style\", \"display:none !important\"), t.removeAttribute(\"class\"), t.innerHTML = \"\") : t.remove(), Y() && (gt(), bt(), et()), oe([document.documentElement, document.body], [p.shown, p[\"height-auto\"], p[\"no-backdrop\"], p[\"toast-shown\"]]) } function en(e) { e = void 0 !== (n = e) ? Object.assign({ isConfirmed: !1, isDenied: !1, isDismissed: !1 }, n) : { isConfirmed: !1, isDenied: !1, isDismissed: !0 }; const t = Gt.swalPromiseResolve.get(this); var n = (e => { const t = g(); if (!t) return false; const n = b.innerParams.get(e); if (!n || $(t, n.hideClass.popup)) return false; oe(t, n.showClass.popup), u(t, n.hideClass.popup); const o = m(); return oe(o, n.showClass.backdrop), u(o, n.hideClass.backdrop), nn(e, t, n), true })(this); this.isAwaitingPromise() ? e.isDismissed || (tn(this), t(e)) : n && t(e) } const tn = e => { e.isAwaitingPromise() && (b.awaitingPromise.delete(e), b.innerParams.get(e) || e._destroy()) }, nn = (e, t, n) => { var o, i, a, r = m(), s = Be && de(t); \"function\" == typeof n.willClose && n.willClose(t), s ? (s = e, o = t, t = r, i = n.returnFocus, a = n.didClose, f.swalCloseEventFinishedCallback = Qt.bind(null, s, t, i, a), o.addEventListener(Be, function (e) { e.target === o && (f.swalCloseEventFinishedCallback(), delete f.swalCloseEventFinishedCallback) })) : Qt(e, r, n.returnFocus, n.didClose) }, on = (e, t) => { setTimeout(() => { \"function\" == typeof t && t.bind(e.params)(), e._destroy() }) }; function an(e, t, n) { const o = b.domCache.get(e); t.forEach(e => { o[e].disabled = n }) } function rn(e, t) { if (!e) return !1; if (\"radio\" === e.type) { const n = e.parentNode.parentNode, o = n.querySelectorAll(\"input\"); for (let e = 0; e < o.length; e++)o[e].disabled = t } else e.disabled = t } const sn = e => { e.isAwaitingPromise() ? (cn(b, e), b.awaitingPromise.set(e, !0)) : (cn(Gt, e), cn(b, e)) }, cn = (e, t) => { for (const n in e) e[n].delete(t) }; var ln = Object.freeze({ hideLoading: $t, disableLoading: $t, getInput: function (e) { var t = b.innerParams.get(e || this); return (e = b.domCache.get(e || this)) ? ee(e.popup, t.input) : null }, close: en, isAwaitingPromise: function () { return !!b.awaitingPromise.get(this) }, rejectPromise: function (e) { const t = Gt.swalPromiseReject.get(this); tn(this), t && t(e) }, closePopup: en, closeModal: en, closeToast: en, enableButtons: function () { an(this, [\"confirmButton\", \"denyButton\", \"cancelButton\"], !1) }, disableButtons: function () { an(this, [\"confirmButton\", \"denyButton\", \"cancelButton\"], !0) }, enableInput: function () { return rn(this.getInput(), !1) }, disableInput: function () { return rn(this.getInput(), !0) }, showValidationMessage: function (e) { const t = b.domCache.get(this); var n = b.innerParams.get(this); l(t.validationMessage, e), t.validationMessage.className = p[\"validation-message\"], n.customClass && n.customClass.validationMessage && u(t.validationMessage, n.customClass.validationMessage), d(t.validationMessage); const o = this.getInput(); o && (o.setAttribute(\"aria-invalid\", !0), o.setAttribute(\"aria-describedby\", p[\"validation-message\"]), te(o), u(o, p.inputerror)) }, resetValidationMessage: function () { var e = b.domCache.get(this); e.validationMessage && h(e.validationMessage); const t = this.getInput(); t && (t.removeAttribute(\"aria-invalid\"), t.removeAttribute(\"aria-describedby\"), oe(t, p.inputerror)) }, getProgressSteps: function () { return b.domCache.get(this).progressSteps }, update: function (e) { var t = g(), n = b.innerParams.get(this); if (!t || $(t, n.hideClass.popup)) return a(\"You're trying to update the closed or closing popup, that won't work. Use the update() method in preConfirm parameter or show a new popup.\"); t = (t => { const n = {}; return Object.keys(t).forEach(e => { if (x(e)) n[e] = t[e]; else a('Invalid parameter to update: \"'.concat(e, '\". Updatable params are listed here: https://github.com/sweetalert2/sweetalert2/blob/master/src/utils/params.js\\n\\nIf you think this parameter should be updatable, request it here: https://github.com/sweetalert2/sweetalert2/issues/new?template=02_feature_request.md')) }), n })(e), n = Object.assign({}, n, t), $e(this, n), b.innerParams.set(this, n), Object.defineProperties(this, { params: { value: Object.assign({}, this.params, e), writable: !1, enumerable: !0 } }) }, _destroy: function () { var e = b.domCache.get(this); const t = b.innerParams.get(this); t ? (e.popup && f.swalCloseEventFinishedCallback && (f.swalCloseEventFinishedCallback(), delete f.swalCloseEventFinishedCallback), f.deferDisposalTimer && (clearTimeout(f.deferDisposalTimer), delete f.deferDisposalTimer), \"function\" == typeof t.didDestroy && t.didDestroy(), e = this, sn(e), delete e.params, delete f.keydownHandler, delete f.keydownTarget, delete f.currentInstance) : sn(this) } }); let un; class dn { constructor() { if (\"undefined\" != typeof window) { un = this; for (var e = arguments.length, t = new Array(e), n = 0; n < e; n++)t[n] = arguments[n]; var o = Object.freeze(this.constructor.argsToParams(t)), o = (Object.defineProperties(this, { params: { value: o, writable: !1, enumerable: !0, configurable: !0 } }), this._main(this.params)); b.promise.set(this, o) } } _main(e) { var t = 1 < arguments.length && void 0 !== arguments[1] ? arguments[1] : {}, e = (T(Object.assign({}, t, e)), f.currentInstance && (f.currentInstance._destroy(), Y() && et()), f.currentInstance = this, mn(e, t)), t = (dt(e), Object.freeze(e), f.timeout && (f.timeout.stop(), delete f.timeout), clearTimeout(f.restoreFocusTimeout), gn(this)); return $e(this, e), b.innerParams.set(this, e), pn(this, t, e) } then(e) { const t = b.promise.get(this); return t.then(e) } finally(e) { const t = b.promise.get(this); return t.finally(e) } } const pn = (l, u, d) => new Promise((e, t) => { const n = e => { l.closePopup({ isDismissed: !0, dismiss: e }) }; var o, i, a; Gt.swalPromiseResolve.set(l, e), Gt.swalPromiseReject.set(l, t), u.confirmButton.onclick = () => { var e = l, t = b.innerParams.get(e); e.disableButtons(), t.input ? St(e, \"confirm\") : Mt(e, !0) }, u.denyButton.onclick = () => { var e = l, t = b.innerParams.get(e); e.disableButtons(), t.returnInputValueOnDeny ? St(e, \"deny\") : Lt(e, !1) }, u.cancelButton.onclick = () => { var e = l, t = n; e.disableButtons(), t(Ge.cancel) }, u.closeButton.onclick = () => n(Ge.close), e = l, t = u, a = n, b.innerParams.get(e).toast ? Dt(e, t, a) : (Ht(t), qt(t), Vt(e, t, a)), o = l, e = f, t = d, i = n, e.keydownTarget && e.keydownHandlerAdded && (e.keydownTarget.removeEventListener(\"keydown\", e.keydownHandler, { capture: e.keydownListenerCapture }), e.keydownHandlerAdded = !1), t.toast || (e.keydownHandler = e => Wt(o, e, i), e.keydownTarget = t.keydownListenerCapture ? window : g(), e.keydownListenerCapture = t.keydownListenerCapture, e.keydownTarget.addEventListener(\"keydown\", e.keydownHandler, { capture: e.keydownListenerCapture }), e.keydownHandlerAdded = !0), a = l, \"select\" === (t = d).input || \"radio\" === t.input ? Pt(a, t) : [\"text\", \"email\", \"number\", \"tel\", \"textarea\"].includes(t.input) && (C(t.inputValue) || A(t.inputValue)) && (At(V()), Bt(a, t)); { var r = d; const s = m(), c = g(); \"function\" == typeof r.willOpen && r.willOpen(c), e = window.getComputedStyle(document.body).overflowY, kt(s, c, r), setTimeout(() => { wt(s, c) }, yt), Y() && (Ct(s, r.scrollbarPadding, e), Qe()), Z() || f.previousActiveElement || (f.previousActiveElement = document.activeElement), \"function\" == typeof r.didOpen && setTimeout(() => r.didOpen(c)), oe(s, p[\"no-transition\"]) } hn(f, d, n), fn(u, d), setTimeout(() => { u.container.scrollTop = 0 }) }), mn = (e, t) => { var n = (e => { e = \"string\" == typeof e.template ? document.querySelector(e.template) : e.template; if (!e) return {}; e = e.content, ct(e), e = Object.assign(nt(e), ot(e), it(e), at(e), rt(e), st(e, tt)); return e })(e); const o = Object.assign({}, r, t, n, e); return o.showClass = Object.assign({}, r.showClass, o.showClass), o.hideClass = Object.assign({}, r.hideClass, o.hideClass), o }, gn = e => { var t = { popup: g(), container: m(), actions: U(), confirmButton: V(), denyButton: N(), cancelButton: F(), loader: R(), closeButton: _(), validationMessage: q(), progressSteps: H() }; return b.domCache.set(e, t), t }, hn = (e, t, n) => { var o = z(); h(o), t.timer && (e.timeout = new pt(() => { n(\"timer\"), delete e.timeout }, t.timer), t.timerProgressBar && (d(o), Q(o, t, \"timerProgressBar\"), setTimeout(() => { e.timeout && e.timeout.running && J(t.timer) }))) }, fn = (e, t) => { if (!t.toast) return w(t.allowEnterKey) ? void (bn(e, t) || Rt(t, -1, 1)) : yn() }, bn = (e, t) => t.focusDeny && ce(e.denyButton) ? (e.denyButton.focus(), !0) : t.focusCancel && ce(e.cancelButton) ? (e.cancelButton.focus(), !0) : !(!t.focusConfirm || !ce(e.confirmButton)) && (e.confirmButton.focus(), !0), yn = () => { document.activeElement instanceof HTMLElement && \"function\" == typeof document.activeElement.blur && document.activeElement.blur() }, vn = (Object.assign(dn.prototype, ln), Object.assign(dn, e), Object.keys(ln).forEach(e => { dn[e] = function () { if (un) return un[e](...arguments) } }), dn.DismissReason = Ge, dn.version = \"11.4.0\", dn); return vn.default = vn, vn }), void 0 !== this && this.Sweetalert2 && (this.swal = this.sweetAlert = this.Swal = this.SweetAlert = this.Sweetalert2);\n</script>\n<script>\n    !function (e, t) { \"object\" == typeof exports && \"undefined\" != typeof module ? module.exports = t() : \"function\" == typeof define && define.amd ? define(t) : (e = e || self).Sweetalert2 = t() }(this, function () { \"use strict\"; const t = \"SweetAlert2:\", y = e => e.charAt(0).toUpperCase() + e.slice(1), i = e => Array.prototype.slice.call(e), a = e => { console.warn(\"\".concat(t, \" \").concat(\"object\" == typeof e ? e.join(\" \") : e)) }, v = e => { console.error(\"\".concat(t, \" \").concat(e)) }, n = [], o = (e, t) => { e = '\"'.concat(e, '\" is deprecated and will be removed in the next major release. Please use \"').concat(t, '\" instead.'), n.includes(e) || (n.push(e), a(e)) }, w = e => \"function\" == typeof e ? e() : e, C = e => e && \"function\" == typeof e.toPromise, k = e => C(e) ? e.toPromise() : Promise.resolve(e), A = e => e && Promise.resolve(e) === e, r = { title: \"\", titleText: \"\", text: \"\", html: \"\", footer: \"\", icon: void 0, iconColor: void 0, iconHtml: void 0, template: void 0, toast: !1, showClass: { popup: \"swal2-show\", backdrop: \"swal2-backdrop-show\", icon: \"swal2-icon-show\" }, hideClass: { popup: \"swal2-hide\", backdrop: \"swal2-backdrop-hide\", icon: \"swal2-icon-hide\" }, customClass: {}, target: \"body\", color: void 0, backdrop: !0, heightAuto: !0, allowOutsideClick: !0, allowEscapeKey: !0, allowEnterKey: !0, stopKeydownPropagation: !0, keydownListenerCapture: !1, showConfirmButton: !0, showDenyButton: !1, showCancelButton: !1, preConfirm: void 0, preDeny: void 0, confirmButtonText: \"OK\", confirmButtonAriaLabel: \"\", confirmButtonColor: void 0, denyButtonText: \"No\", denyButtonAriaLabel: \"\", denyButtonColor: void 0, cancelButtonText: \"Cancel\", cancelButtonAriaLabel: \"\", cancelButtonColor: void 0, buttonsStyling: !0, reverseButtons: !1, focusConfirm: !0, focusDeny: !1, focusCancel: !1, returnFocus: !0, showCloseButton: !1, closeButtonHtml: \"&times;\", closeButtonAriaLabel: \"Close this dialog\", loaderHtml: \"\", showLoaderOnConfirm: !1, showLoaderOnDeny: !1, imageUrl: void 0, imageWidth: void 0, imageHeight: void 0, imageAlt: \"\", timer: void 0, timerProgressBar: !1, width: void 0, padding: void 0, background: void 0, input: void 0, inputPlaceholder: \"\", inputLabel: \"\", inputValue: \"\", inputOptions: {}, inputAutoTrim: !0, inputAttributes: {}, inputValidator: void 0, returnInputValueOnDeny: !1, validationMessage: void 0, grow: !1, position: \"center\", progressSteps: [], currentProgressStep: void 0, progressStepsDistance: void 0, willOpen: void 0, didOpen: void 0, didRender: void 0, willClose: void 0, didClose: void 0, didDestroy: void 0, scrollbarPadding: !0 }, s = [\"allowEscapeKey\", \"allowOutsideClick\", \"background\", \"buttonsStyling\", \"cancelButtonAriaLabel\", \"cancelButtonColor\", \"cancelButtonText\", \"closeButtonAriaLabel\", \"closeButtonHtml\", \"color\", \"confirmButtonAriaLabel\", \"confirmButtonColor\", \"confirmButtonText\", \"currentProgressStep\", \"customClass\", \"denyButtonAriaLabel\", \"denyButtonColor\", \"denyButtonText\", \"didClose\", \"didDestroy\", \"footer\", \"hideClass\", \"html\", \"icon\", \"iconColor\", \"iconHtml\", \"imageAlt\", \"imageHeight\", \"imageUrl\", \"imageWidth\", \"preConfirm\", \"preDeny\", \"progressSteps\", \"returnFocus\", \"reverseButtons\", \"showCancelButton\", \"showCloseButton\", \"showConfirmButton\", \"showDenyButton\", \"text\", \"title\", \"titleText\", \"willClose\"], c = {}, P = [\"allowOutsideClick\", \"allowEnterKey\", \"backdrop\", \"focusConfirm\", \"focusDeny\", \"focusCancel\", \"returnFocus\", \"heightAuto\", \"keydownListenerCapture\"], B = e => Object.prototype.hasOwnProperty.call(r, e), x = e => -1 !== s.indexOf(e), E = e => c[e], T = e => { !e.backdrop && e.allowOutsideClick && a('\"allowOutsideClick\" parameter requires `backdrop` parameter to be set to `true`'); for (const n in e) t = n, B(t) || a('Unknown parameter \"'.concat(t, '\"')), e.toast && (t = n, P.includes(t) && a('The parameter \"'.concat(t, '\" is incompatible with toasts'))), t = n, E(t) && o(t, E(t)); var t }; var e = e => { const t = {}; for (const n in e) t[e[n]] = \"swal2-\" + e[n]; return t }; const p = e([\"container\", \"shown\", \"height-auto\", \"iosfix\", \"popup\", \"modal\", \"no-backdrop\", \"no-transition\", \"toast\", \"toast-shown\", \"show\", \"hide\", \"close\", \"title\", \"html-container\", \"actions\", \"confirm\", \"deny\", \"cancel\", \"default-outline\", \"footer\", \"icon\", \"icon-content\", \"image\", \"input\", \"file\", \"range\", \"select\", \"radio\", \"checkbox\", \"label\", \"textarea\", \"inputerror\", \"input-label\", \"validation-message\", \"progress-steps\", \"active-progress-step\", \"progress-step\", \"progress-step-line\", \"loader\", \"loading\", \"styled\", \"top\", \"top-start\", \"top-end\", \"top-left\", \"top-right\", \"center\", \"center-start\", \"center-end\", \"center-left\", \"center-right\", \"bottom\", \"bottom-start\", \"bottom-end\", \"bottom-left\", \"bottom-right\", \"grow-row\", \"grow-column\", \"grow-fullscreen\", \"rtl\", \"timer-progress-bar\", \"timer-progress-bar-container\", \"scrollbar-measure\", \"icon-success\", \"icon-warning\", \"icon-info\", \"icon-question\", \"icon-error\"]), S = e([\"success\", \"warning\", \"info\", \"question\", \"error\"]), m = () => document.body.querySelector(\".\".concat(p.container)), L = e => { const t = m(); return t ? t.querySelector(e) : null }, O = e => L(\".\".concat(e)), g = () => O(p.popup), j = () => O(p.icon), M = () => O(p.title), D = () => O(p[\"html-container\"]), I = () => O(p.image), H = () => O(p[\"progress-steps\"]), q = () => O(p[\"validation-message\"]), V = () => L(\".\".concat(p.actions, \" .\").concat(p.confirm)), N = () => L(\".\".concat(p.actions, \" .\").concat(p.deny)); const R = () => L(\".\".concat(p.loader)), F = () => L(\".\".concat(p.actions, \" .\").concat(p.cancel)), U = () => O(p.actions), W = () => O(p.footer), z = () => O(p[\"timer-progress-bar\"]), _ = () => O(p.close), K = () => { const e = i(g().querySelectorAll('[tabindex]:not([tabindex=\"-1\"]):not([tabindex=\"0\"])')).sort((e, t) => { e = parseInt(e.getAttribute(\"tabindex\")), t = parseInt(t.getAttribute(\"tabindex\")); return t < e ? 1 : e < t ? -1 : 0 }); var t = i(g().querySelectorAll('\\n  a[href],\\n  area[href],\\n  input:not([disabled]),\\n  select:not([disabled]),\\n  textarea:not([disabled]),\\n  button:not([disabled]),\\n  iframe,\\n  object,\\n  embed,\\n  [tabindex=\"0\"],\\n  [contenteditable],\\n  audio[controls],\\n  video[controls],\\n  summary\\n')).filter(e => \"-1\" !== e.getAttribute(\"tabindex\")); return (t => { const n = []; for (let e = 0; e < t.length; e++)-1 === n.indexOf(t[e]) && n.push(t[e]); return n })(e.concat(t)).filter(e => ce(e)) }, Y = () => !$(document.body, p[\"toast-shown\"]) && !$(document.body, p[\"no-backdrop\"]), Z = () => g() && $(g(), p.toast); function J(e) { var t = 1 < arguments.length && void 0 !== arguments[1] && arguments[1]; const n = z(); ce(n) && (t && (n.style.transition = \"none\", n.style.width = \"100%\"), setTimeout(() => { n.style.transition = \"width \".concat(e / 1e3, \"s linear\"), n.style.width = \"0%\" }, 10)) } const X = { previousBodyPadding: null }, l = (t, e) => { if (t.textContent = \"\", e) { const n = new DOMParser, o = n.parseFromString(e, \"text/html\"); i(o.querySelector(\"head\").childNodes).forEach(e => { t.appendChild(e) }), i(o.querySelector(\"body\").childNodes).forEach(e => { t.appendChild(e) }) } }, $ = (t, e) => { if (!e) return !1; var n = e.split(/\\s+/); for (let e = 0; e < n.length; e++)if (!t.classList.contains(n[e])) return !1; return !0 }, G = (t, n) => { i(t.classList).forEach(e => { Object.values(p).includes(e) || Object.values(S).includes(e) || Object.values(n.showClass).includes(e) || t.classList.remove(e) }) }, Q = (e, t, n) => { if (G(e, t), t.customClass && t.customClass[n]) { if (\"string\" != typeof t.customClass[n] && !t.customClass[n].forEach) return a(\"Invalid type of customClass.\".concat(n, '! Expected string or iterable object, got \"').concat(typeof t.customClass[n], '\"')); u(e, t.customClass[n]) } }, ee = (e, t) => { if (!t) return null; switch (t) { case \"select\": case \"textarea\": case \"file\": return e.querySelector(\".\".concat(p.popup, \" > .\").concat(p[t])); case \"checkbox\": return e.querySelector(\".\".concat(p.popup, \" > .\").concat(p.checkbox, \" input\")); case \"radio\": return e.querySelector(\".\".concat(p.popup, \" > .\").concat(p.radio, \" input:checked\")) || e.querySelector(\".\".concat(p.popup, \" > .\").concat(p.radio, \" input:first-child\")); case \"range\": return e.querySelector(\".\".concat(p.popup, \" > .\").concat(p.range, \" input\")); default: return e.querySelector(\".\".concat(p.popup, \" > .\").concat(p.input)) } }, te = e => { var t; e.focus(), \"file\" !== e.type && (t = e.value, e.value = \"\", e.value = t) }, ne = (e, t, n) => { e && t && (t = \"string\" == typeof t ? t.split(/\\s+/).filter(Boolean) : t).forEach(t => { Array.isArray(e) ? e.forEach(e => { n ? e.classList.add(t) : e.classList.remove(t) }) : n ? e.classList.add(t) : e.classList.remove(t) }) }, u = (e, t) => { ne(e, t, !0) }, oe = (e, t) => { ne(e, t, !1) }, ie = (e, t) => { var n = i(e.childNodes); for (let e = 0; e < n.length; e++)if ($(n[e], t)) return n[e] }, ae = (e, t, n) => { (n = n === \"\".concat(parseInt(n)) ? parseInt(n) : n) || 0 === parseInt(n) ? e.style[t] = \"number\" == typeof n ? \"\".concat(n, \"px\") : n : e.style.removeProperty(t) }, d = function (e) { e.style.display = 1 < arguments.length && void 0 !== arguments[1] ? arguments[1] : \"flex\" }, h = e => { e.style.display = \"none\" }, re = (e, t, n, o) => { const i = e.querySelector(t); i && (i.style[n] = o) }, se = (e, t, n) => { t ? d(e, n) : h(e) }, ce = e => !(!e || !(e.offsetWidth || e.offsetHeight || e.getClientRects().length)), le = () => !ce(V()) && !ce(N()) && !ce(F()), ue = e => !!(e.scrollHeight > e.clientHeight), de = e => { const t = window.getComputedStyle(e); var e = parseFloat(t.getPropertyValue(\"animation-duration\") || \"0\"), n = parseFloat(t.getPropertyValue(\"transition-duration\") || \"0\"); return 0 < e || 0 < n }, pe = () => \"undefined\" == typeof window || \"undefined\" == typeof document, me = 100, f = {}, ge = () => { f.previousActiveElement && f.previousActiveElement.focus ? (f.previousActiveElement.focus(), f.previousActiveElement = null) : document.body && document.body.focus() }, he = o => new Promise(e => { if (!o) return e(); var t = window.scrollX, n = window.scrollY; f.restoreFocusTimeout = setTimeout(() => { ge(), e() }, me), window.scrollTo(t, n) }), fe = '\\n <div aria-labelledby=\"'.concat(p.title, '\" aria-describedby=\"').concat(p[\"html-container\"], '\" class=\"').concat(p.popup, '\" tabindex=\"-1\">\\n   <button type=\"button\" class=\"').concat(p.close, '\"></button>\\n   <ul class=\"').concat(p[\"progress-steps\"], '\"></ul>\\n   <div class=\"').concat(p.icon, '\"></div>\\n   <img class=\"').concat(p.image, '\" />\\n   <h2 class=\"').concat(p.title, '\" id=\"').concat(p.title, '\"></h2>\\n   <div class=\"').concat(p[\"html-container\"], '\" id=\"').concat(p[\"html-container\"], '\"></div>\\n   <input class=\"').concat(p.input, '\" />\\n   <input type=\"file\" class=\"').concat(p.file, '\" />\\n   <div class=\"').concat(p.range, '\">\\n     <input type=\"range\" />\\n     <output></output>\\n   </div>\\n   <select class=\"').concat(p.select, '\"></select>\\n   <div class=\"').concat(p.radio, '\"></div>\\n   <label for=\"').concat(p.checkbox, '\" class=\"').concat(p.checkbox, '\">\\n     <input type=\"checkbox\" />\\n     <span class=\"').concat(p.label, '\"></span>\\n   </label>\\n   <textarea class=\"').concat(p.textarea, '\"></textarea>\\n   <div class=\"').concat(p[\"validation-message\"], '\" id=\"').concat(p[\"validation-message\"], '\"></div>\\n   <div class=\"').concat(p.actions, '\">\\n     <div class=\"').concat(p.loader, '\"></div>\\n     <button type=\"button\" class=\"').concat(p.confirm, '\"></button>\\n     <button type=\"button\" class=\"').concat(p.deny, '\"></button>\\n     <button type=\"button\" class=\"').concat(p.cancel, '\"></button>\\n   </div>\\n   <div class=\"').concat(p.footer, '\"></div>\\n   <div class=\"').concat(p[\"timer-progress-bar-container\"], '\">\\n     <div class=\"').concat(p[\"timer-progress-bar\"], '\"></div>\\n   </div>\\n </div>\\n').replace(/(^|\\n)\\s*/g, \"\"), be = () => { const e = m(); return !!e && (e.remove(), oe([document.documentElement, document.body], [p[\"no-backdrop\"], p[\"toast-shown\"], p[\"has-column\"]]), !0) }, ye = () => { f.currentInstance.resetValidationMessage() }, ve = () => { const e = g(), t = ie(e, p.input), n = ie(e, p.file), o = e.querySelector(\".\".concat(p.range, \" input\")), i = e.querySelector(\".\".concat(p.range, \" output\")), a = ie(e, p.select), r = e.querySelector(\".\".concat(p.checkbox, \" input\")), s = ie(e, p.textarea); t.oninput = ye, n.onchange = ye, a.onchange = ye, r.onchange = ye, s.oninput = ye, o.oninput = () => { ye(), i.value = o.value }, o.onchange = () => { ye(), o.nextSibling.value = o.value } }, we = e => \"string\" == typeof e ? document.querySelector(e) : e, Ce = e => { const t = g(); t.setAttribute(\"role\", e.toast ? \"alert\" : \"dialog\"), t.setAttribute(\"aria-live\", e.toast ? \"polite\" : \"assertive\"), e.toast || t.setAttribute(\"aria-modal\", \"true\") }, ke = e => { \"rtl\" === window.getComputedStyle(e).direction && u(m(), p.rtl) }, Ae = (e, t) => { if (e instanceof HTMLElement) t.appendChild(e); else if (\"object\" == typeof e) { var n = e, o = t; if (n.jquery) Pe(o, n); else l(o, n.toString()) } else e && l(t, e) }, Pe = (t, n) => { if (t.textContent = \"\", 0 in n) for (let e = 0; e in n; e++)t.appendChild(n[e].cloneNode(!0)); else t.appendChild(n.cloneNode(!0)) }, Be = (() => { if (pe()) return !1; var e = document.createElement(\"div\"), t = { WebkitAnimation: \"webkitAnimationEnd\", animation: \"animationend\" }; for (const n in t) if (Object.prototype.hasOwnProperty.call(t, n) && void 0 !== e.style[n]) return t[n]; return !1 })(), xe = (e, t) => { var n, o, i, a, r, s = U(), c = R(); (t.showConfirmButton || t.showDenyButton || t.showCancelButton ? d : h)(s), Q(s, t, \"actions\"), s = s, n = c, o = t, i = V(), a = N(), r = F(), Ee(i, \"confirm\", o), Ee(a, \"deny\", o), Ee(r, \"cancel\", o), function (e, t, n, o) { if (!o.buttonsStyling) return oe([e, t, n], p.styled); u([e, t, n], p.styled), o.confirmButtonColor && (e.style.backgroundColor = o.confirmButtonColor, u(e, p[\"default-outline\"])); o.denyButtonColor && (t.style.backgroundColor = o.denyButtonColor, u(t, p[\"default-outline\"])); o.cancelButtonColor && (n.style.backgroundColor = o.cancelButtonColor, u(n, p[\"default-outline\"])) }(i, a, r, o), o.reverseButtons && (o.toast ? (s.insertBefore(r, i), s.insertBefore(a, i)) : (s.insertBefore(r, n), s.insertBefore(a, n), s.insertBefore(i, n))), l(c, t.loaderHtml), Q(c, t, \"loader\") }; function Ee(e, t, n) { se(e, n[\"show\".concat(y(t), \"Button\")], \"inline-block\"), l(e, n[\"\".concat(t, \"ButtonText\")]), e.setAttribute(\"aria-label\", n[\"\".concat(t, \"ButtonAriaLabel\")]), e.className = p[t], Q(e, n, \"\".concat(t, \"Button\")), u(e, n[\"\".concat(t, \"ButtonClass\")]) } const Te = (e, t) => { var n, o, i = m(); i && (o = i, \"string\" == typeof (n = t.backdrop) ? o.style.background = n : n || u([document.documentElement, document.body], p[\"no-backdrop\"]), o = i, (n = t.position) in p ? u(o, p[n]) : (a('The \"position\" parameter is not valid, defaulting to \"center\"'), u(o, p.center)), n = i, !(o = t.grow) || \"string\" != typeof o || (o = \"grow-\".concat(o)) in p && u(n, p[o]), Q(i, t, \"container\")) }; var b = { awaitingPromise: new WeakMap, promise: new WeakMap, innerParams: new WeakMap, domCache: new WeakMap }; const Se = [\"input\", \"file\", \"range\", \"select\", \"radio\", \"checkbox\", \"textarea\"], Le = (e, r) => { const s = g(); var t, e = b.innerParams.get(e); const c = !e || r.input !== e.input; Se.forEach(e => { var t = p[e]; const n = ie(s, t); { var o = r.inputAttributes; const i = ee(g(), e); if (i) { Oe(i); for (const a in o) i.setAttribute(a, o[a]) } } n.className = t, c && h(n) }), r.input && (c && (e => { if (!Ie[e.input]) return v('Unexpected type of input! Expected \"text\", \"email\", \"password\", \"number\", \"tel\", \"select\", \"radio\", \"checkbox\", \"textarea\", \"file\" or \"url\", got \"'.concat(e.input, '\"')); const t = De(e.input), n = Ie[e.input](t, e); d(n), setTimeout(() => { te(n) }) })(r), e = r, t = De(e.input), e.customClass && u(t, e.customClass.input)) }, Oe = t => { for (let e = 0; e < t.attributes.length; e++) { var n = t.attributes[e].name;[\"type\", \"value\", \"style\"].includes(n) || t.removeAttribute(n) } }, je = (e, t) => { e.placeholder && !t.inputPlaceholder || (e.placeholder = t.inputPlaceholder) }, Me = (e, t, n) => { if (n.inputLabel) { e.id = p.input; const i = document.createElement(\"label\"); var o = p[\"input-label\"]; i.setAttribute(\"for\", e.id), i.className = o, u(i, n.customClass.inputLabel), i.innerText = n.inputLabel, t.insertAdjacentElement(\"beforebegin\", i) } }, De = e => { e = p[e] || p.input; return ie(g(), e) }, Ie = {}, He = (Ie.text = Ie.email = Ie.password = Ie.number = Ie.tel = Ie.url = (e, t) => (\"string\" == typeof t.inputValue || \"number\" == typeof t.inputValue ? e.value = t.inputValue : A(t.inputValue) || a('Unexpected type of inputValue! Expected \"string\", \"number\" or \"Promise\", got \"'.concat(typeof t.inputValue, '\"')), Me(e, e, t), je(e, t), e.type = t.input, e), Ie.file = (e, t) => (Me(e, e, t), je(e, t), e), Ie.range = (e, t) => { const n = e.querySelector(\"input\"), o = e.querySelector(\"output\"); return n.value = t.inputValue, n.type = t.input, o.value = t.inputValue, Me(n, e, t), e }, Ie.select = (e, t) => { if (e.textContent = \"\", t.inputPlaceholder) { const n = document.createElement(\"option\"); l(n, t.inputPlaceholder), n.value = \"\", n.disabled = !0, n.selected = !0, e.appendChild(n) } return Me(e, e, t), e }, Ie.radio = e => (e.textContent = \"\", e), Ie.checkbox = (e, t) => { const n = ee(g(), \"checkbox\"); n.value = \"1\", n.id = p.checkbox, n.checked = Boolean(t.inputValue); var o = e.querySelector(\"span\"); return l(o, t.inputPlaceholder), e }, Ie.textarea = (n, e) => { n.value = e.inputValue, je(n, e), Me(n, n, e); return setTimeout(() => { if (\"MutationObserver\" in window) { const t = parseInt(window.getComputedStyle(g()).width); new MutationObserver(() => { var e = n.offsetWidth + (e = n, parseInt(window.getComputedStyle(e).marginLeft) + parseInt(window.getComputedStyle(e).marginRight)); e > t ? g().style.width = \"\".concat(e, \"px\") : g().style.width = null }).observe(n, { attributes: !0, attributeFilter: [\"style\"] }) } }), n }, (e, t) => { const n = D(); Q(n, t, \"htmlContainer\"), t.html ? (Ae(t.html, n), d(n, \"block\")) : t.text ? (n.textContent = t.text, d(n, \"block\")) : h(n), Le(e, t) }), qe = (e, t) => { var n = W(); se(n, t.footer), t.footer && Ae(t.footer, n), Q(n, t, \"footer\") }, Ve = (e, t) => { const n = _(); l(n, t.closeButtonHtml), Q(n, t, \"closeButton\"), se(n, t.showCloseButton), n.setAttribute(\"aria-label\", t.closeButtonAriaLabel) }, Ne = (e, t) => { var e = b.innerParams.get(e), n = j(); return e && t.icon === e.icon ? (ze(n, t), void Re(n, t)) : t.icon || t.iconHtml ? t.icon && -1 === Object.keys(S).indexOf(t.icon) ? (v('Unknown icon! Expected \"success\", \"error\", \"warning\", \"info\" or \"question\", got \"'.concat(t.icon, '\"')), h(n)) : (d(n), ze(n, t), Re(n, t), void u(n, t.showClass.icon)) : h(n) }, Re = (e, t) => { for (const n in S) t.icon !== n && oe(e, S[n]); u(e, S[t.icon]), _e(e, t), Fe(), Q(e, t, \"icon\") }, Fe = () => { const e = g(); var t = window.getComputedStyle(e).getPropertyValue(\"background-color\"); const n = e.querySelectorAll(\"[class^=swal2-success-circular-line], .swal2-success-fix\"); for (let e = 0; e < n.length; e++)n[e].style.backgroundColor = t }, Ue = '\\n  <div class=\"swal2-success-circular-line-left\"></div>\\n  <span class=\"swal2-success-line-tip\"></span> <span class=\"swal2-success-line-long\"></span>\\n  <div class=\"swal2-success-ring\"></div> <div class=\"swal2-success-fix\"></div>\\n  <div class=\"swal2-success-circular-line-right\"></div>\\n', We = '\\n  <span class=\"swal2-x-mark\">\\n    <span class=\"swal2-x-mark-line-left\"></span>\\n    <span class=\"swal2-x-mark-line-right\"></span>\\n  </span>\\n', ze = (e, t) => { var n; e.textContent = \"\", t.iconHtml ? l(e, Ke(t.iconHtml)) : \"success\" === t.icon ? l(e, Ue) : \"error\" === t.icon ? l(e, We) : (n = { question: \"?\", warning: \"!\", info: \"i\" }, l(e, Ke(n[t.icon]))) }, _e = (e, t) => { if (t.iconColor) { e.style.color = t.iconColor, e.style.borderColor = t.iconColor; for (const n of [\".swal2-success-line-tip\", \".swal2-success-line-long\", \".swal2-x-mark-line-left\", \".swal2-x-mark-line-right\"]) re(e, n, \"backgroundColor\", t.iconColor); re(e, \".swal2-success-ring\", \"borderColor\", t.iconColor) } }, Ke = e => '<div class=\"'.concat(p[\"icon-content\"], '\">').concat(e, \"</div>\"), Ye = (e, t) => { const n = I(); if (!t.imageUrl) return h(n); d(n, \"\"), n.setAttribute(\"src\", t.imageUrl), n.setAttribute(\"alt\", t.imageAlt), ae(n, \"width\", t.imageWidth), ae(n, \"height\", t.imageHeight), n.className = p.image, Q(n, t, \"image\") }, Ze = (e, o) => { const i = H(); if (!o.progressSteps || 0 === o.progressSteps.length) return h(i); d(i), i.textContent = \"\", o.currentProgressStep >= o.progressSteps.length && a(\"Invalid currentProgressStep parameter, it should be less than progressSteps.length (currentProgressStep like JS arrays starts from 0)\"), o.progressSteps.forEach((e, t) => { e = e, n = document.createElement(\"li\"), u(n, p[\"progress-step\"]), l(n, e); var n, e = n; i.appendChild(e), t === o.currentProgressStep && u(e, p[\"active-progress-step\"]), t !== o.progressSteps.length - 1 && (n = (e => { const t = document.createElement(\"li\"); return u(t, p[\"progress-step-line\"]), e.progressStepsDistance && (t.style.width = e.progressStepsDistance), t })(o), i.appendChild(n)) }) }, Je = (e, t) => { const n = M(); se(n, t.title || t.titleText, \"block\"), t.title && Ae(t.title, n), t.titleText && (n.innerText = t.titleText), Q(n, t, \"title\") }, Xe = (e, t) => { var n = m(); const o = g(); t.toast ? (ae(n, \"width\", t.width), o.style.width = \"100%\", o.insertBefore(R(), j())) : ae(o, \"width\", t.width), ae(o, \"padding\", t.padding), t.color && (o.style.color = t.color), t.background && (o.style.background = t.background), h(q()); n = o; (n.className = \"\".concat(p.popup, \" \").concat(ce(n) ? t.showClass.popup : \"\"), t.toast) ? (u([document.documentElement, document.body], p[\"toast-shown\"]), u(n, p.toast)) : u(n, p.modal); Q(n, t, \"popup\"), \"string\" == typeof t.customClass && u(n, t.customClass); t.icon && u(n, p[\"icon-\".concat(t.icon)]) }, $e = (e, t) => { Xe(e, t), Te(e, t), Ze(e, t), Ne(e, t), Ye(e, t), Je(e, t), Ve(e, t), He(e, t), xe(e, t), qe(e, t), \"function\" == typeof t.didRender && t.didRender(g()) }, Ge = Object.freeze({ cancel: \"cancel\", backdrop: \"backdrop\", close: \"close\", esc: \"esc\", timer: \"timer\" }), Qe = () => { const e = i(document.body.children); e.forEach(e => { e === m() || e.contains(m()) || (e.hasAttribute(\"aria-hidden\") && e.setAttribute(\"data-previous-aria-hidden\", e.getAttribute(\"aria-hidden\")), e.setAttribute(\"aria-hidden\", \"true\")) }) }, et = () => { const e = i(document.body.children); e.forEach(e => { e.hasAttribute(\"data-previous-aria-hidden\") ? (e.setAttribute(\"aria-hidden\", e.getAttribute(\"data-previous-aria-hidden\")), e.removeAttribute(\"data-previous-aria-hidden\")) : e.removeAttribute(\"aria-hidden\") }) }, tt = [\"swal-title\", \"swal-html\", \"swal-footer\"], nt = e => { const n = {}; return i(e.querySelectorAll(\"swal-param\")).forEach(e => { lt(e, [\"name\", \"value\"]); var t = e.getAttribute(\"name\"), e = e.getAttribute(\"value\"); \"boolean\" == typeof r[t] && \"false\" === e && (n[t] = !1), \"object\" == typeof r[t] && (n[t] = JSON.parse(e)) }), n }, ot = e => { const n = {}; return i(e.querySelectorAll(\"swal-button\")).forEach(e => { lt(e, [\"type\", \"color\", \"aria-label\"]); var t = e.getAttribute(\"type\"); n[\"\".concat(t, \"ButtonText\")] = e.innerHTML, n[\"show\".concat(y(t), \"Button\")] = !0, e.hasAttribute(\"color\") && (n[\"\".concat(t, \"ButtonColor\")] = e.getAttribute(\"color\")), e.hasAttribute(\"aria-label\") && (n[\"\".concat(t, \"ButtonAriaLabel\")] = e.getAttribute(\"aria-label\")) }), n }, it = e => { const t = {}, n = e.querySelector(\"swal-image\"); return n && (lt(n, [\"src\", \"width\", \"height\", \"alt\"]), n.hasAttribute(\"src\") && (t.imageUrl = n.getAttribute(\"src\")), n.hasAttribute(\"width\") && (t.imageWidth = n.getAttribute(\"width\")), n.hasAttribute(\"height\") && (t.imageHeight = n.getAttribute(\"height\")), n.hasAttribute(\"alt\") && (t.imageAlt = n.getAttribute(\"alt\"))), t }, at = e => { const t = {}, n = e.querySelector(\"swal-icon\"); return n && (lt(n, [\"type\", \"color\"]), n.hasAttribute(\"type\") && (t.icon = n.getAttribute(\"type\")), n.hasAttribute(\"color\") && (t.iconColor = n.getAttribute(\"color\")), t.iconHtml = n.innerHTML), t }, rt = e => { const n = {}, t = e.querySelector(\"swal-input\"); t && (lt(t, [\"type\", \"label\", \"placeholder\", \"value\"]), n.input = t.getAttribute(\"type\") || \"text\", t.hasAttribute(\"label\") && (n.inputLabel = t.getAttribute(\"label\")), t.hasAttribute(\"placeholder\") && (n.inputPlaceholder = t.getAttribute(\"placeholder\")), t.hasAttribute(\"value\") && (n.inputValue = t.getAttribute(\"value\"))); e = e.querySelectorAll(\"swal-input-option\"); return e.length && (n.inputOptions = {}, i(e).forEach(e => { lt(e, [\"value\"]); var t = e.getAttribute(\"value\"), e = e.innerHTML; n.inputOptions[t] = e })), n }, st = (e, t) => { const n = {}; for (const o in t) { const i = t[o], a = e.querySelector(i); a && (lt(a, []), n[i.replace(/^swal-/, \"\")] = a.innerHTML.trim()) } return n }, ct = e => { const t = tt.concat([\"swal-param\", \"swal-button\", \"swal-image\", \"swal-icon\", \"swal-input\", \"swal-input-option\"]); i(e.children).forEach(e => { e = e.tagName.toLowerCase(); -1 === t.indexOf(e) && a(\"Unrecognized element <\".concat(e, \">\")) }) }, lt = (t, n) => { i(t.attributes).forEach(e => { -1 === n.indexOf(e.name) && a(['Unrecognized attribute \"'.concat(e.name, '\" on <').concat(t.tagName.toLowerCase(), \">.\"), \"\".concat(n.length ? \"Allowed attributes are: \".concat(n.join(\", \")) : \"To set the value, use HTML within the element.\")]) }) }; var ut = { email: (e, t) => /^[a-zA-Z0-9.+_-]+@[a-zA-Z0-9.-]+\\.[a-zA-Z0-9-]{2,24}$/.test(e) ? Promise.resolve() : Promise.resolve(t || \"Invalid email address\"), url: (e, t) => /^https?:\\/\\/(www\\.)?[-a-zA-Z0-9@:%._+~#=]{1,256}\\.[a-z]{2,63}\\b([-a-zA-Z0-9@:%_+.~#?&/=]*)$/.test(e) ? Promise.resolve() : Promise.resolve(t || \"Invalid URL\") }; function dt(e) { (t = e).inputValidator || Object.keys(ut).forEach(e => { t.input === e && (t.inputValidator = ut[e]) }), e.showLoaderOnConfirm && !e.preConfirm && a(\"showLoaderOnConfirm is set to true, but preConfirm is not defined.\\nshowLoaderOnConfirm should be used together with preConfirm, see usage example:\\nhttps://sweetalert2.github.io/#ajax-request\"), (n = e).target && (\"string\" != typeof n.target || document.querySelector(n.target)) && (\"string\" == typeof n.target || n.target.appendChild) || (a('Target parameter is not valid, defaulting to \"body\"'), n.target = \"body\"), \"string\" == typeof e.title && (e.title = e.title.split(\"\\n\").join(\"<br />\")); var t, n = e, e = be(); if (pe()) v(\"SweetAlert2 requires document to initialize\"); else { const o = document.createElement(\"div\"), i = (o.className = p.container, e && u(o, p[\"no-transition\"]), l(o, fe), we(n.target)); i.appendChild(o), Ce(n), ke(i), ve() } } class pt { constructor(e, t) { this.callback = e, this.remaining = t, this.running = !1, this.start() } start() { return this.running || (this.running = !0, this.started = new Date, this.id = setTimeout(this.callback, this.remaining)), this.remaining } stop() { return this.running && (this.running = !1, clearTimeout(this.id), this.remaining -= (new Date).getTime() - this.started.getTime()), this.remaining } increase(e) { var t = this.running; return t && this.stop(), this.remaining += e, t && this.start(), this.remaining } getTimerLeft() { return this.running && (this.stop(), this.start()), this.remaining } isRunning() { return this.running } } const mt = () => { null === X.previousBodyPadding && document.body.scrollHeight > window.innerHeight && (X.previousBodyPadding = parseInt(window.getComputedStyle(document.body).getPropertyValue(\"padding-right\")), document.body.style.paddingRight = \"\".concat(X.previousBodyPadding + (() => { const e = document.createElement(\"div\"); e.className = p[\"scrollbar-measure\"], document.body.appendChild(e); var t = e.getBoundingClientRect().width - e.clientWidth; return document.body.removeChild(e), t })(), \"px\")) }, gt = () => { null !== X.previousBodyPadding && (document.body.style.paddingRight = \"\".concat(X.previousBodyPadding, \"px\"), X.previousBodyPadding = null) }, ht = () => { var e = /iPad|iPhone|iPod/.test(navigator.userAgent) && !window.MSStream || \"MacIntel\" === navigator.platform && 1 < navigator.maxTouchPoints; if (e && !$(document.body, p.iosfix)) { var t, e = document.body.scrollTop; document.body.style.top = \"\".concat(-1 * e, \"px\"), u(document.body, p.iosfix); { const n = m(); let t; n.ontouchstart = e => { t = ft(e) }, n.ontouchmove = e => { t && (e.preventDefault(), e.stopPropagation()) } } { const o = navigator.userAgent, i = !!o.match(/iPad/i) || !!o.match(/iPhone/i), a = !!o.match(/WebKit/i), r = i && a && !o.match(/CriOS/i); r && (t = 44, g().scrollHeight > window.innerHeight - 44 && (m().style.paddingBottom = \"\".concat(44, \"px\"))) } } }, ft = e => { var t, n = e.target, o = m(); return !((t = e).touches && t.touches.length && \"stylus\" === t.touches[0].touchType || (t = e).touches && 1 < t.touches.length) && (n === o || !(ue(o) || \"INPUT\" === n.tagName || \"TEXTAREA\" === n.tagName || ue(D()) && D().contains(n))) }, bt = () => { var e; $(document.body, p.iosfix) && (e = parseInt(document.body.style.top, 10), oe(document.body, p.iosfix), document.body.style.top = \"\", document.body.scrollTop = -1 * e) }, yt = 10, vt = e => { const t = g(); if (e.target === t) { const n = m(); t.removeEventListener(Be, vt), n.style.overflowY = \"auto\" } }, wt = (e, t) => { Be && de(t) ? (e.style.overflowY = \"hidden\", t.addEventListener(Be, vt)) : e.style.overflowY = \"auto\" }, Ct = (e, t, n) => { ht(), t && \"hidden\" !== n && mt(), setTimeout(() => { e.scrollTop = 0 }) }, kt = (e, t, n) => { u(e, n.showClass.backdrop), t.style.setProperty(\"opacity\", \"0\", \"important\"), d(t, \"grid\"), setTimeout(() => { u(t, n.showClass.popup), t.style.removeProperty(\"opacity\") }, yt), u([document.documentElement, document.body], p.shown), n.heightAuto && n.backdrop && !n.toast && u([document.documentElement, document.body], p[\"height-auto\"]) }, At = e => { let t = g(); t || new vn, t = g(); var n = R(); if (Z()) h(j()); else { var o = t; const i = U(), a = R(); !e && ce(V()) && (e = V()); d(i), e && (h(e), a.setAttribute(\"data-button-to-replace\", e.className)); a.parentNode.insertBefore(a, e), u([o, i], p.loading) } d(n), t.setAttribute(\"data-loading\", !0), t.setAttribute(\"aria-busy\", !0), t.focus() }, Pt = (t, n) => { const o = g(), i = e => xt[n.input](o, Et(e), n); C(n.inputOptions) || A(n.inputOptions) ? (At(V()), k(n.inputOptions).then(e => { t.hideLoading(), i(e) })) : \"object\" == typeof n.inputOptions ? i(n.inputOptions) : v(\"Unexpected type of inputOptions! Expected object, Map or Promise, got \".concat(typeof n.inputOptions)) }, Bt = (t, n) => { const o = t.getInput(); h(o), k(n.inputValue).then(e => { o.value = \"number\" === n.input ? parseFloat(e) || 0 : \"\".concat(e), d(o), o.focus(), t.hideLoading() }).catch(e => { v(\"Error in inputValue promise: \".concat(e)), o.value = \"\", d(o), o.focus(), t.hideLoading() }) }, xt = { select: (e, t, i) => { const a = ie(e, p.select), r = (e, t, n) => { const o = document.createElement(\"option\"); o.value = n, l(o, t), o.selected = Tt(n, i.inputValue), e.appendChild(o) }; t.forEach(e => { var t = e[0]; const n = e[1]; if (Array.isArray(n)) { const o = document.createElement(\"optgroup\"); o.label = t, o.disabled = !1, a.appendChild(o), n.forEach(e => r(o, e[1], e[0])) } else r(a, n, t) }), a.focus() }, radio: (e, t, a) => { const r = ie(e, p.radio), n = (t.forEach(e => { var t = e[0], e = e[1]; const n = document.createElement(\"input\"), o = document.createElement(\"label\"), i = (n.type = \"radio\", n.name = p.radio, n.value = t, Tt(t, a.inputValue) && (n.checked = !0), document.createElement(\"span\")); l(i, e), i.className = p.label, o.appendChild(n), o.appendChild(i), r.appendChild(o) }), r.querySelectorAll(\"input\")); n.length && n[0].focus() } }, Et = n => { const o = []; return \"undefined\" != typeof Map && n instanceof Map ? n.forEach((e, t) => { let n = e; \"object\" == typeof n && (n = Et(n)), o.push([t, n]) }) : Object.keys(n).forEach(e => { let t = n[e]; \"object\" == typeof t && (t = Et(t)), o.push([e, t]) }), o }, Tt = (e, t) => t && t.toString() === e.toString(), St = (e, t) => { var n = b.innerParams.get(e); if (!n.input) return v('The \"input\" parameter is needed to be set when using returnInputValueOn'.concat(y(t))); var o = ((e, t) => { const n = e.getInput(); if (!n) return null; switch (t.input) { case \"checkbox\": return n.checked ? 1 : 0; case \"radio\": return (o = n).checked ? o.value : null; case \"file\": return (o = n).files.length ? null !== o.getAttribute(\"multiple\") ? o.files : o.files[0] : null; default: return t.inputAutoTrim ? n.value.trim() : n.value }var o })(e, n); if (n.inputValidator) { var i = e; var a = o; var r = t; const s = b.innerParams.get(i), c = (i.disableInput(), Promise.resolve().then(() => k(s.inputValidator(a, s.validationMessage)))); c.then(e => { i.enableButtons(), i.enableInput(), e ? i.showValidationMessage(e) : (\"deny\" === r ? Lt : Mt)(i, a) }) } else e.getInput().checkValidity() ? (\"deny\" === t ? Lt : Mt)(e, o) : (e.enableButtons(), e.showValidationMessage(n.validationMessage)) }, Lt = (t, n) => { const e = b.innerParams.get(t || void 0); if (e.showLoaderOnDeny && At(N()), e.preDeny) { b.awaitingPromise.set(t || void 0, !0); const o = Promise.resolve().then(() => k(e.preDeny(n, e.validationMessage))); o.then(e => { !1 === e ? t.hideLoading() : t.closePopup({ isDenied: !0, value: void 0 === e ? n : e }) }).catch(e => jt(t || void 0, e)) } else t.closePopup({ isDenied: !0, value: n }) }, Ot = (e, t) => { e.closePopup({ isConfirmed: !0, value: t }) }, jt = (e, t) => { e.rejectPromise(t) }, Mt = (t, n) => { const e = b.innerParams.get(t || void 0); if (e.showLoaderOnConfirm && At(), e.preConfirm) { t.resetValidationMessage(), b.awaitingPromise.set(t || void 0, !0); const o = Promise.resolve().then(() => k(e.preConfirm(n, e.validationMessage))); o.then(e => { ce(q()) || !1 === e ? t.hideLoading() : Ot(t, void 0 === e ? n : e) }).catch(e => jt(t || void 0, e)) } else Ot(t, n) }, Dt = (n, e, o) => { e.popup.onclick = () => { var e, t = b.innerParams.get(n); t && ((e = t).showConfirmButton || e.showDenyButton || e.showCancelButton || e.showCloseButton || t.timer || t.input) || o(Ge.close) } }; let It = !1; const Ht = t => { t.popup.onmousedown = () => { t.container.onmouseup = function (e) { t.container.onmouseup = void 0, e.target === t.container && (It = !0) } } }, qt = t => { t.container.onmousedown = () => { t.popup.onmouseup = function (e) { t.popup.onmouseup = void 0, e.target !== t.popup && !t.popup.contains(e.target) || (It = !0) } } }, Vt = (n, o, i) => { o.container.onclick = e => { var t = b.innerParams.get(n); It ? It = !1 : e.target === o.container && w(t.allowOutsideClick) && i(Ge.backdrop) } }; const Nt = () => V() && V().click(); const Rt = (e, t, n) => { const o = K(); if (o.length) return (t += n) === o.length ? t = 0 : -1 === t && (t = o.length - 1), o[t].focus(); g().focus() }, Ft = [\"ArrowRight\", \"ArrowDown\"], Ut = [\"ArrowLeft\", \"ArrowUp\"], Wt = (e, n, o) => { var i = b.innerParams.get(e); if (i) if (i.stopKeydownPropagation && n.stopPropagation(), \"Enter\" === n.key) e = e, a = n, t = i, w(t.allowEnterKey) && !a.isComposing && a.target && e.getInput() && a.target.outerHTML === e.getInput().outerHTML && ([\"textarea\", \"file\"].includes(t.input) || (Nt(), a.preventDefault())); else if (\"Tab\" !== n.key) { if ([...Ft, ...Ut].includes(n.key)) { e = n.key; const s = V(), c = N(), d = F(); if ([s, c, d].includes(document.activeElement)) { var t = Ft.includes(e) ? \"nextElementSibling\" : \"previousElementSibling\"; const l = document.activeElement[t]; l instanceof HTMLElement && l.focus() } } else if (\"Escape\" === n.key) { var a = n, e = i; if (w(e.allowEscapeKey)) { a.preventDefault(); o(Ge.esc) } } } else { e = n; o = i; var u = e.target, r = K(); let t = -1; for (let e = 0; e < r.length; e++)if (u === r[e]) { t = e; break } e.shiftKey ? Rt(o, t, -1) : Rt(o, t, 1); e.stopPropagation(), e.preventDefault() } }, zt = e => \"object\" == typeof e && e.jquery, _t = e => e instanceof Element || zt(e); const Kt = () => { if (f.timeout) { { const n = z(); var e = parseInt(window.getComputedStyle(n).width), t = (n.style.removeProperty(\"transition\"), n.style.width = \"100%\", parseInt(window.getComputedStyle(n).width)), e = e / t * 100; n.style.removeProperty(\"transition\"), n.style.width = \"\".concat(e, \"%\") } return f.timeout.stop() } }, Yt = () => { var e; if (f.timeout) return e = f.timeout.start(), J(e), e }; let Zt = !1; const Jt = {}; const Xt = t => { for (let e = t.target; e && e !== document; e = e.parentNode)for (const o in Jt) { var n = e.getAttribute(o); if (n) return void Jt[o].fire({ template: n }) } }; e = Object.freeze({ isValidParameter: B, isUpdatableParameter: x, isDeprecatedParameter: E, argsToParams: n => { const o = {}; return \"object\" != typeof n[0] || _t(n[0]) ? [\"title\", \"html\", \"icon\"].forEach((e, t) => { t = n[t]; \"string\" == typeof t || _t(t) ? o[e] = t : void 0 !== t && v(\"Unexpected type of \".concat(e, '! Expected \"string\" or \"Element\", got ').concat(typeof t)) }) : Object.assign(o, n[0]), o }, isVisible: () => ce(g()), clickConfirm: Nt, clickDeny: () => N() && N().click(), clickCancel: () => F() && F().click(), getContainer: m, getPopup: g, getTitle: M, getHtmlContainer: D, getImage: I, getIcon: j, getInputLabel: () => O(p[\"input-label\"]), getCloseButton: _, getActions: U, getConfirmButton: V, getDenyButton: N, getCancelButton: F, getLoader: R, getFooter: W, getTimerProgressBar: z, getFocusableElements: K, getValidationMessage: q, isLoading: () => g().hasAttribute(\"data-loading\"), fire: function () { for (var e = arguments.length, t = new Array(e), n = 0; n < e; n++)t[n] = arguments[n]; return new this(...t) }, mixin: function (n) { class e extends this{ _main(e, t) { return super._main(e, Object.assign({}, n, t)) } } return e }, showLoading: At, enableLoading: At, getTimerLeft: () => f.timeout && f.timeout.getTimerLeft(), stopTimer: Kt, resumeTimer: Yt, toggleTimer: () => { var e = f.timeout; return e && (e.running ? Kt : Yt)() }, increaseTimer: e => { if (f.timeout) return e = f.timeout.increase(e), J(e, !0), e }, isTimerRunning: () => f.timeout && f.timeout.isRunning(), bindClickHandler: function () { var e = 0 < arguments.length && void 0 !== arguments[0] ? arguments[0] : \"data-swal-template\"; Jt[e] = this, Zt || (document.body.addEventListener(\"click\", Xt), Zt = !0) } }); function $t() { var e, t = b.innerParams.get(this); if (t) { const n = b.domCache.get(this); h(n.loader), Z() ? t.icon && d(j()) : (t = n, (e = t.popup.getElementsByClassName(t.loader.getAttribute(\"data-button-to-replace\"))).length ? d(e[0], \"inline-block\") : le() && h(t.actions)), oe([n.popup, n.actions], p.loading), n.popup.removeAttribute(\"aria-busy\"), n.popup.removeAttribute(\"data-loading\"), n.confirmButton.disabled = !1, n.denyButton.disabled = !1, n.cancelButton.disabled = !1 } } var Gt = { swalPromiseResolve: new WeakMap, swalPromiseReject: new WeakMap }; function Qt(e, t, n, o) { Z() ? on(e, o) : (he(n).then(() => on(e, o)), f.keydownTarget.removeEventListener(\"keydown\", f.keydownHandler, { capture: f.keydownListenerCapture }), f.keydownHandlerAdded = !1), /^((?!chrome|android).)*safari/i.test(navigator.userAgent) ? (t.setAttribute(\"style\", \"display:none !important\"), t.removeAttribute(\"class\"), t.innerHTML = \"\") : t.remove(), Y() && (gt(), bt(), et()), oe([document.documentElement, document.body], [p.shown, p[\"height-auto\"], p[\"no-backdrop\"], p[\"toast-shown\"]]) } function en(e) { e = void 0 !== (n = e) ? Object.assign({ isConfirmed: !1, isDenied: !1, isDismissed: !1 }, n) : { isConfirmed: !1, isDenied: !1, isDismissed: !0 }; const t = Gt.swalPromiseResolve.get(this); var n = (e => { const t = g(); if (!t) return false; const n = b.innerParams.get(e); if (!n || $(t, n.hideClass.popup)) return false; oe(t, n.showClass.popup), u(t, n.hideClass.popup); const o = m(); return oe(o, n.showClass.backdrop), u(o, n.hideClass.backdrop), nn(e, t, n), true })(this); this.isAwaitingPromise() ? e.isDismissed || (tn(this), t(e)) : n && t(e) } const tn = e => { e.isAwaitingPromise() && (b.awaitingPromise.delete(e), b.innerParams.get(e) || e._destroy()) }, nn = (e, t, n) => { var o, i, a, r = m(), s = Be && de(t); \"function\" == typeof n.willClose && n.willClose(t), s ? (s = e, o = t, t = r, i = n.returnFocus, a = n.didClose, f.swalCloseEventFinishedCallback = Qt.bind(null, s, t, i, a), o.addEventListener(Be, function (e) { e.target === o && (f.swalCloseEventFinishedCallback(), delete f.swalCloseEventFinishedCallback) })) : Qt(e, r, n.returnFocus, n.didClose) }, on = (e, t) => { setTimeout(() => { \"function\" == typeof t && t.bind(e.params)(), e._destroy() }) }; function an(e, t, n) { const o = b.domCache.get(e); t.forEach(e => { o[e].disabled = n }) } function rn(e, t) { if (!e) return !1; if (\"radio\" === e.type) { const n = e.parentNode.parentNode, o = n.querySelectorAll(\"input\"); for (let e = 0; e < o.length; e++)o[e].disabled = t } else e.disabled = t } const sn = e => { e.isAwaitingPromise() ? (cn(b, e), b.awaitingPromise.set(e, !0)) : (cn(Gt, e), cn(b, e)) }, cn = (e, t) => { for (const n in e) e[n].delete(t) }; var ln = Object.freeze({ hideLoading: $t, disableLoading: $t, getInput: function (e) { var t = b.innerParams.get(e || this); return (e = b.domCache.get(e || this)) ? ee(e.popup, t.input) : null }, close: en, isAwaitingPromise: function () { return !!b.awaitingPromise.get(this) }, rejectPromise: function (e) { const t = Gt.swalPromiseReject.get(this); tn(this), t && t(e) }, closePopup: en, closeModal: en, closeToast: en, enableButtons: function () { an(this, [\"confirmButton\", \"denyButton\", \"cancelButton\"], !1) }, disableButtons: function () { an(this, [\"confirmButton\", \"denyButton\", \"cancelButton\"], !0) }, enableInput: function () { return rn(this.getInput(), !1) }, disableInput: function () { return rn(this.getInput(), !0) }, showValidationMessage: function (e) { const t = b.domCache.get(this); var n = b.innerParams.get(this); l(t.validationMessage, e), t.validationMessage.className = p[\"validation-message\"], n.customClass && n.customClass.validationMessage && u(t.validationMessage, n.customClass.validationMessage), d(t.validationMessage); const o = this.getInput(); o && (o.setAttribute(\"aria-invalid\", !0), o.setAttribute(\"aria-describedby\", p[\"validation-message\"]), te(o), u(o, p.inputerror)) }, resetValidationMessage: function () { var e = b.domCache.get(this); e.validationMessage && h(e.validationMessage); const t = this.getInput(); t && (t.removeAttribute(\"aria-invalid\"), t.removeAttribute(\"aria-describedby\"), oe(t, p.inputerror)) }, getProgressSteps: function () { return b.domCache.get(this).progressSteps }, update: function (e) { var t = g(), n = b.innerParams.get(this); if (!t || $(t, n.hideClass.popup)) return a(\"You're trying to update the closed or closing popup, that won't work. Use the update() method in preConfirm parameter or show a new popup.\"); t = (t => { const n = {}; return Object.keys(t).forEach(e => { if (x(e)) n[e] = t[e]; else a('Invalid parameter to update: \"'.concat(e, '\". Updatable params are listed here: https://github.com/sweetalert2/sweetalert2/blob/master/src/utils/params.js\\n\\nIf you think this parameter should be updatable, request it here: https://github.com/sweetalert2/sweetalert2/issues/new?template=02_feature_request.md')) }), n })(e), n = Object.assign({}, n, t), $e(this, n), b.innerParams.set(this, n), Object.defineProperties(this, { params: { value: Object.assign({}, this.params, e), writable: !1, enumerable: !0 } }) }, _destroy: function () { var e = b.domCache.get(this); const t = b.innerParams.get(this); t ? (e.popup && f.swalCloseEventFinishedCallback && (f.swalCloseEventFinishedCallback(), delete f.swalCloseEventFinishedCallback), f.deferDisposalTimer && (clearTimeout(f.deferDisposalTimer), delete f.deferDisposalTimer), \"function\" == typeof t.didDestroy && t.didDestroy(), e = this, sn(e), delete e.params, delete f.keydownHandler, delete f.keydownTarget, delete f.currentInstance) : sn(this) } }); let un; class dn { constructor() { if (\"undefined\" != typeof window) { un = this; for (var e = arguments.length, t = new Array(e), n = 0; n < e; n++)t[n] = arguments[n]; var o = Object.freeze(this.constructor.argsToParams(t)), o = (Object.defineProperties(this, { params: { value: o, writable: !1, enumerable: !0, configurable: !0 } }), this._main(this.params)); b.promise.set(this, o) } } _main(e) { var t = 1 < arguments.length && void 0 !== arguments[1] ? arguments[1] : {}, e = (T(Object.assign({}, t, e)), f.currentInstance && (f.currentInstance._destroy(), Y() && et()), f.currentInstance = this, mn(e, t)), t = (dt(e), Object.freeze(e), f.timeout && (f.timeout.stop(), delete f.timeout), clearTimeout(f.restoreFocusTimeout), gn(this)); return $e(this, e), b.innerParams.set(this, e), pn(this, t, e) } then(e) { const t = b.promise.get(this); return t.then(e) } finally(e) { const t = b.promise.get(this); return t.finally(e) } } const pn = (l, u, d) => new Promise((e, t) => { const n = e => { l.closePopup({ isDismissed: !0, dismiss: e }) }; var o, i, a; Gt.swalPromiseResolve.set(l, e), Gt.swalPromiseReject.set(l, t), u.confirmButton.onclick = () => { var e = l, t = b.innerParams.get(e); e.disableButtons(), t.input ? St(e, \"confirm\") : Mt(e, !0) }, u.denyButton.onclick = () => { var e = l, t = b.innerParams.get(e); e.disableButtons(), t.returnInputValueOnDeny ? St(e, \"deny\") : Lt(e, !1) }, u.cancelButton.onclick = () => { var e = l, t = n; e.disableButtons(), t(Ge.cancel) }, u.closeButton.onclick = () => n(Ge.close), e = l, t = u, a = n, b.innerParams.get(e).toast ? Dt(e, t, a) : (Ht(t), qt(t), Vt(e, t, a)), o = l, e = f, t = d, i = n, e.keydownTarget && e.keydownHandlerAdded && (e.keydownTarget.removeEventListener(\"keydown\", e.keydownHandler, { capture: e.keydownListenerCapture }), e.keydownHandlerAdded = !1), t.toast || (e.keydownHandler = e => Wt(o, e, i), e.keydownTarget = t.keydownListenerCapture ? window : g(), e.keydownListenerCapture = t.keydownListenerCapture, e.keydownTarget.addEventListener(\"keydown\", e.keydownHandler, { capture: e.keydownListenerCapture }), e.keydownHandlerAdded = !0), a = l, \"select\" === (t = d).input || \"radio\" === t.input ? Pt(a, t) : [\"text\", \"email\", \"number\", \"tel\", \"textarea\"].includes(t.input) && (C(t.inputValue) || A(t.inputValue)) && (At(V()), Bt(a, t)); { var r = d; const s = m(), c = g(); \"function\" == typeof r.willOpen && r.willOpen(c), e = window.getComputedStyle(document.body).overflowY, kt(s, c, r), setTimeout(() => { wt(s, c) }, yt), Y() && (Ct(s, r.scrollbarPadding, e), Qe()), Z() || f.previousActiveElement || (f.previousActiveElement = document.activeElement), \"function\" == typeof r.didOpen && setTimeout(() => r.didOpen(c)), oe(s, p[\"no-transition\"]) } hn(f, d, n), fn(u, d), setTimeout(() => { u.container.scrollTop = 0 }) }), mn = (e, t) => { var n = (e => { e = \"string\" == typeof e.template ? document.querySelector(e.template) : e.template; if (!e) return {}; e = e.content, ct(e), e = Object.assign(nt(e), ot(e), it(e), at(e), rt(e), st(e, tt)); return e })(e); const o = Object.assign({}, r, t, n, e); return o.showClass = Object.assign({}, r.showClass, o.showClass), o.hideClass = Object.assign({}, r.hideClass, o.hideClass), o }, gn = e => { var t = { popup: g(), container: m(), actions: U(), confirmButton: V(), denyButton: N(), cancelButton: F(), loader: R(), closeButton: _(), validationMessage: q(), progressSteps: H() }; return b.domCache.set(e, t), t }, hn = (e, t, n) => { var o = z(); h(o), t.timer && (e.timeout = new pt(() => { n(\"timer\"), delete e.timeout }, t.timer), t.timerProgressBar && (d(o), Q(o, t, \"timerProgressBar\"), setTimeout(() => { e.timeout && e.timeout.running && J(t.timer) }))) }, fn = (e, t) => { if (!t.toast) return w(t.allowEnterKey) ? void (bn(e, t) || Rt(t, -1, 1)) : yn() }, bn = (e, t) => t.focusDeny && ce(e.denyButton) ? (e.denyButton.focus(), !0) : t.focusCancel && ce(e.cancelButton) ? (e.cancelButton.focus(), !0) : !(!t.focusConfirm || !ce(e.confirmButton)) && (e.confirmButton.focus(), !0), yn = () => { document.activeElement instanceof HTMLElement && \"function\" == typeof document.activeElement.blur && document.activeElement.blur() }, vn = (Object.assign(dn.prototype, ln), Object.assign(dn, e), Object.keys(ln).forEach(e => { dn[e] = function () { if (un) return un[e](...arguments) } }), dn.DismissReason = Ge, dn.version = \"11.4.0\", dn); return vn.default = vn, vn }), void 0 !== this && this.Sweetalert2 && (this.swal = this.sweetAlert = this.Swal = this.SweetAlert = this.Sweetalert2);\n</script>\n<style>\n    .swal2-popup.swal2-toast {\n        box-sizing: border-box;\n        grid-column: 1/4 !important;\n        grid-row: 1/4 !important;\n        grid-template-columns: 1fr 99fr 1fr;\n        padding: 1em;\n        overflow-y: hidden;\n        background: #fff;\n        box-shadow: 0 0 1px rgba(0, 0, 0, .075), 0 1px 2px rgba(0, 0, 0, .075), 1px 2px 4px rgba(0, 0, 0, .075), 1px 3px 8px rgba(0, 0, 0, .075), 2px 4px 16px rgba(0, 0, 0, .075);\n        pointer-events: all\n    }\n\n    .swal2-popup.swal2-toast>* {\n        grid-column: 2\n    }\n\n    .swal2-popup.swal2-toast .swal2-title {\n        margin: .5em 1em;\n        padding: 0;\n        font-size: 1em;\n        text-align: initial\n    }\n\n    .swal2-popup.swal2-toast .swal2-loading {\n        justify-content: center\n    }\n\n    .swal2-popup.swal2-toast .swal2-input {\n        height: 2em;\n        margin: .5em;\n        font-size: 1em\n    }\n\n    .swal2-popup.swal2-toast .swal2-validation-message {\n        font-size: 1em\n    }\n\n    .swal2-popup.swal2-toast .swal2-footer {\n        margin: .5em 0 0;\n        padding: .5em 0 0;\n        font-size: .8em\n    }\n\n    .swal2-popup.swal2-toast .swal2-close {\n        grid-column: 3/3;\n        grid-row: 1/99;\n        align-self: center;\n        width: .8em;\n        height: .8em;\n        margin: 0;\n        font-size: 2em\n    }\n\n    .swal2-popup.swal2-toast .swal2-html-container {\n        margin: .5em 1em;\n        padding: 0;\n        font-size: 1em;\n        text-align: initial\n    }\n\n    .swal2-popup.swal2-toast .swal2-html-container:empty {\n        padding: 0\n    }\n\n    .swal2-popup.swal2-toast .swal2-loader {\n        grid-column: 1;\n        grid-row: 1/99;\n        align-self: center;\n        width: 2em;\n        height: 2em;\n        margin: .25em\n    }\n\n    .swal2-popup.swal2-toast .swal2-icon {\n        grid-column: 1;\n        grid-row: 1/99;\n        align-self: center;\n        width: 2em;\n        min-width: 2em;\n        height: 2em;\n        margin: 0 .5em 0 0\n    }\n\n    .swal2-popup.swal2-toast .swal2-icon .swal2-icon-content {\n        display: flex;\n        align-items: center;\n        font-size: 1.8em;\n        font-weight: 700\n    }\n\n    .swal2-popup.swal2-toast .swal2-icon.swal2-success .swal2-success-ring {\n        width: 2em;\n        height: 2em\n    }\n\n    .swal2-popup.swal2-toast .swal2-icon.swal2-error [class^=swal2-x-mark-line] {\n        top: .875em;\n        width: 1.375em\n    }\n\n    .swal2-popup.swal2-toast .swal2-icon.swal2-error [class^=swal2-x-mark-line][class$=left] {\n        left: .3125em\n    }\n\n    .swal2-popup.swal2-toast .swal2-icon.swal2-error [class^=swal2-x-mark-line][class$=right] {\n        right: .3125em\n    }\n\n    .swal2-popup.swal2-toast .swal2-actions {\n        justify-content: flex-start;\n        height: auto;\n        margin: 0;\n        margin-top: .5em;\n        padding: 0 .5em\n    }\n\n    .swal2-popup.swal2-toast .swal2-styled {\n        margin: .25em .5em;\n        padding: .4em .6em;\n        font-size: 1em\n    }\n\n    .swal2-popup.swal2-toast .swal2-success {\n        border-color: #a5dc86\n    }\n\n    .swal2-popup.swal2-toast .swal2-success [class^=swal2-success-circular-line] {\n        position: absolute;\n        width: 1.6em;\n        height: 3em;\n        transform: rotate(45deg);\n        border-radius: 50%\n    }\n\n    .swal2-popup.swal2-toast .swal2-success [class^=swal2-success-circular-line][class$=left] {\n        top: -.8em;\n        left: -.5em;\n        transform: rotate(-45deg);\n        transform-origin: 2em 2em;\n        border-radius: 4em 0 0 4em\n    }\n\n    .swal2-popup.swal2-toast .swal2-success [class^=swal2-success-circular-line][class$=right] {\n        top: -.25em;\n        left: .9375em;\n        transform-origin: 0 1.5em;\n        border-radius: 0 4em 4em 0\n    }\n\n    .swal2-popup.swal2-toast .swal2-success .swal2-success-ring {\n        width: 2em;\n        height: 2em\n    }\n\n    .swal2-popup.swal2-toast .swal2-success .swal2-success-fix {\n        top: 0;\n        left: .4375em;\n        width: .4375em;\n        height: 2.6875em\n    }\n\n    .swal2-popup.swal2-toast .swal2-success [class^=swal2-success-line] {\n        height: .3125em\n    }\n\n    .swal2-popup.swal2-toast .swal2-success [class^=swal2-success-line][class$=tip] {\n        top: 1.125em;\n        left: .1875em;\n        width: .75em\n    }\n\n    .swal2-popup.swal2-toast .swal2-success [class^=swal2-success-line][class$=long] {\n        top: .9375em;\n        right: .1875em;\n        width: 1.375em\n    }\n\n    .swal2-popup.swal2-toast .swal2-success.swal2-icon-show .swal2-success-line-tip {\n        -webkit-animation: swal2-toast-animate-success-line-tip .75s;\n        animation: swal2-toast-animate-success-line-tip .75s\n    }\n\n    .swal2-popup.swal2-toast .swal2-success.swal2-icon-show .swal2-success-line-long {\n        -webkit-animation: swal2-toast-animate-success-line-long .75s;\n        animation: swal2-toast-animate-success-line-long .75s\n    }\n\n    .swal2-popup.swal2-toast.swal2-show {\n        -webkit-animation: swal2-toast-show .5s;\n        animation: swal2-toast-show .5s\n    }\n\n    .swal2-popup.swal2-toast.swal2-hide {\n        -webkit-animation: swal2-toast-hide .1s forwards;\n        animation: swal2-toast-hide .1s forwards\n    }\n\n    .swal2-container {\n        display: grid;\n        position: fixed;\n        z-index: 1060;\n        top: 0;\n        right: 0;\n        bottom: 0;\n        left: 0;\n        box-sizing: border-box;\n        grid-template-areas: \"top-start     top            top-end\"\"center-start  center         center-end\"\"bottom-start  bottom-center  bottom-end\";\n        grid-template-rows: minmax(-webkit-min-content, auto) minmax(-webkit-min-content, auto) minmax(-webkit-min-content, auto);\n        grid-template-rows: minmax(min-content, auto) minmax(min-content, auto) minmax(min-content, auto);\n        height: 100%;\n        padding: .625em;\n        overflow-x: hidden;\n        transition: background-color .1s;\n        -webkit-overflow-scrolling: touch\n    }\n\n    .swal2-container.swal2-backdrop-show,\n    .swal2-container.swal2-noanimation {\n        background: rgba(0, 0, 0, .4)\n    }\n\n    .swal2-container.swal2-backdrop-hide {\n        background: 0 0 !important\n    }\n\n    .swal2-container.swal2-bottom-start,\n    .swal2-container.swal2-center-start,\n    .swal2-container.swal2-top-start {\n        grid-template-columns: minmax(0, 1fr) auto auto\n    }\n\n    .swal2-container.swal2-bottom,\n    .swal2-container.swal2-center,\n    .swal2-container.swal2-top {\n        grid-template-columns: auto minmax(0, 1fr) auto\n    }\n\n    .swal2-container.swal2-bottom-end,\n    .swal2-container.swal2-center-end,\n    .swal2-container.swal2-top-end {\n        grid-template-columns: auto auto minmax(0, 1fr)\n    }\n\n    .swal2-container.swal2-top-start>.swal2-popup {\n        align-self: start\n    }\n\n    .swal2-container.swal2-top>.swal2-popup {\n        grid-column: 2;\n        align-self: start;\n        justify-self: center\n    }\n\n    .swal2-container.swal2-top-end>.swal2-popup,\n    .swal2-container.swal2-top-right>.swal2-popup {\n        grid-column: 3;\n        align-self: start;\n        justify-self: end\n    }\n\n    .swal2-container.swal2-center-left>.swal2-popup,\n    .swal2-container.swal2-center-start>.swal2-popup {\n        grid-row: 2;\n        align-self: center\n    }\n\n    .swal2-container.swal2-center>.swal2-popup {\n        grid-column: 2;\n        grid-row: 2;\n        align-self: center;\n        justify-self: center\n    }\n\n    .swal2-container.swal2-center-end>.swal2-popup,\n    .swal2-container.swal2-center-right>.swal2-popup {\n        grid-column: 3;\n        grid-row: 2;\n        align-self: center;\n        justify-self: end\n    }\n\n    .swal2-container.swal2-bottom-left>.swal2-popup,\n    .swal2-container.swal2-bottom-start>.swal2-popup {\n        grid-column: 1;\n        grid-row: 3;\n        align-self: end\n    }\n\n    .swal2-container.swal2-bottom>.swal2-popup {\n        grid-column: 2;\n        grid-row: 3;\n        justify-self: center;\n        align-self: end\n    }\n\n    .swal2-container.swal2-bottom-end>.swal2-popup,\n    .swal2-container.swal2-bottom-right>.swal2-popup {\n        grid-column: 3;\n        grid-row: 3;\n        align-self: end;\n        justify-self: end\n    }\n\n    .swal2-container.swal2-grow-fullscreen>.swal2-popup,\n    .swal2-container.swal2-grow-row>.swal2-popup {\n        grid-column: 1/4;\n        width: 100%\n    }\n\n    .swal2-container.swal2-grow-column>.swal2-popup,\n    .swal2-container.swal2-grow-fullscreen>.swal2-popup {\n        grid-row: 1/4;\n        align-self: stretch\n    }\n\n    .swal2-container.swal2-no-transition {\n        transition: none !important\n    }\n\n    .swal2-popup {\n        display: none;\n        position: relative;\n        box-sizing: border-box;\n        grid-template-columns: minmax(0, 100%);\n        width: 32em;\n        max-width: 100%;\n        padding: 0 0 1.25em;\n        border: none;\n        border-radius: 5px;\n        background: #fff;\n        color: #545454;\n        font-family: inherit;\n        font-size: 1rem\n    }\n\n    .swal2-popup:focus {\n        outline: 0\n    }\n\n    .swal2-popup.swal2-loading {\n        overflow-y: hidden\n    }\n\n    .swal2-title {\n        position: relative;\n        max-width: 100%;\n        margin: 0;\n        padding: .8em 1em 0;\n        color: inherit;\n        font-size: 1.875em;\n        font-weight: 600;\n        text-align: center;\n        text-transform: none;\n        word-wrap: break-word\n    }\n\n    .swal2-actions {\n        display: flex;\n        z-index: 1;\n        box-sizing: border-box;\n        flex-wrap: wrap;\n        align-items: center;\n        justify-content: center;\n        width: auto;\n        margin: 1.25em auto 0;\n        padding: 0\n    }\n\n    .swal2-actions:not(.swal2-loading) .swal2-styled[disabled] {\n        opacity: .4\n    }\n\n    .swal2-actions:not(.swal2-loading) .swal2-styled:hover {\n        background-image: linear-gradient(rgba(0, 0, 0, .1), rgba(0, 0, 0, .1))\n    }\n\n    .swal2-actions:not(.swal2-loading) .swal2-styled:active {\n        background-image: linear-gradient(rgba(0, 0, 0, .2), rgba(0, 0, 0, .2))\n    }\n\n    .swal2-loader {\n        display: none;\n        align-items: center;\n        justify-content: center;\n        width: 2.2em;\n        height: 2.2em;\n        margin: 0 1.875em;\n        -webkit-animation: swal2-rotate-loading 1.5s linear 0s infinite normal;\n        animation: swal2-rotate-loading 1.5s linear 0s infinite normal;\n        border-width: .25em;\n        border-style: solid;\n        border-radius: 100%;\n        border-color: #2778c4 transparent #2778c4 transparent\n    }\n\n    .swal2-styled {\n        margin: .3125em;\n        padding: .625em 1.1em;\n        transition: box-shadow .1s;\n        box-shadow: 0 0 0 3px transparent;\n        font-weight: 500\n    }\n\n    .swal2-styled:not([disabled]) {\n        cursor: pointer\n    }\n\n    .swal2-styled.swal2-confirm {\n        border: 0;\n        border-radius: .25em;\n        background: initial;\n        background-color: #7066e0;\n        color: #fff;\n        font-size: 1em\n    }\n\n    .swal2-styled.swal2-confirm:focus {\n        box-shadow: 0 0 0 3px rgba(112, 102, 224, .5)\n    }\n\n    .swal2-styled.swal2-deny {\n        border: 0;\n        border-radius: .25em;\n        background: initial;\n        background-color: #dc3741;\n        color: #fff;\n        font-size: 1em\n    }\n\n    .swal2-styled.swal2-deny:focus {\n        box-shadow: 0 0 0 3px rgba(220, 55, 65, .5)\n    }\n\n    .swal2-styled.swal2-cancel {\n        border: 0;\n        border-radius: .25em;\n        background: initial;\n        background-color: #6e7881;\n        color: #fff;\n        font-size: 1em\n    }\n\n    .swal2-styled.swal2-cancel:focus {\n        box-shadow: 0 0 0 3px rgba(110, 120, 129, .5)\n    }\n\n    .swal2-styled.swal2-default-outline:focus {\n        box-shadow: 0 0 0 3px rgba(100, 150, 200, .5)\n    }\n\n    .swal2-styled:focus {\n        outline: 0\n    }\n\n    .swal2-styled::-moz-focus-inner {\n        border: 0\n    }\n\n    .swal2-footer {\n        justify-content: center;\n        margin: 1em 0 0;\n        padding: 1em 1em 0;\n        border-top: 1px solid #eee;\n        color: inherit;\n        font-size: 1em\n    }\n\n    .swal2-timer-progress-bar-container {\n        position: absolute;\n        right: 0;\n        bottom: 0;\n        left: 0;\n        grid-column: auto !important;\n        overflow: hidden;\n        border-bottom-right-radius: 5px;\n        border-bottom-left-radius: 5px\n    }\n\n    .swal2-timer-progress-bar {\n        width: 100%;\n        height: .25em;\n        background: rgba(0, 0, 0, .2)\n    }\n\n    .swal2-image {\n        max-width: 100%;\n        margin: 2em auto 1em\n    }\n\n    .swal2-close {\n        z-index: 2;\n        align-items: center;\n        justify-content: center;\n        width: 1.2em;\n        height: 1.2em;\n        margin-top: 0;\n        margin-right: 0;\n        margin-bottom: -1.2em;\n        padding: 0;\n        overflow: hidden;\n        transition: color .1s, box-shadow .1s;\n        border: none;\n        border-radius: 5px;\n        background: 0 0;\n        color: #ccc;\n        font-family: serif;\n        font-family: monospace;\n        font-size: 2.5em;\n        cursor: pointer;\n        justify-self: end\n    }\n\n    .swal2-close:hover {\n        transform: none;\n        background: 0 0;\n        color: #f27474\n    }\n\n    .swal2-close:focus {\n        outline: 0;\n        box-shadow: inset 0 0 0 3px rgba(100, 150, 200, .5)\n    }\n\n    .swal2-close::-moz-focus-inner {\n        border: 0\n    }\n\n    .swal2-html-container {\n        z-index: 1;\n        justify-content: center;\n        margin: 1em 1.6em .3em;\n        padding: 0;\n        overflow: auto;\n        color: inherit;\n        font-size: 1.125em;\n        font-weight: 400;\n        line-height: normal;\n        text-align: center;\n        word-wrap: break-word;\n        word-break: break-word\n    }\n\n    .swal2-checkbox,\n    .swal2-file,\n    .swal2-input,\n    .swal2-radio,\n    .swal2-select,\n    .swal2-textarea {\n        margin: 1em 2em 3px\n    }\n\n    .swal2-file,\n    .swal2-input,\n    .swal2-textarea {\n        box-sizing: border-box;\n        width: auto;\n        transition: border-color .1s, box-shadow .1s;\n        border: 1px solid #d9d9d9;\n        border-radius: .1875em;\n        background: inherit;\n        box-shadow: inset 0 1px 1px rgba(0, 0, 0, .06), 0 0 0 3px transparent;\n        color: inherit;\n        font-size: 1.125em\n    }\n\n    .swal2-file.swal2-inputerror,\n    .swal2-input.swal2-inputerror,\n    .swal2-textarea.swal2-inputerror {\n        border-color: #f27474 !important;\n        box-shadow: 0 0 2px #f27474 !important\n    }\n\n    .swal2-file:focus,\n    .swal2-input:focus,\n    .swal2-textarea:focus {\n        border: 1px solid #b4dbed;\n        outline: 0;\n        box-shadow: inset 0 1px 1px rgba(0, 0, 0, .06), 0 0 0 3px rgba(100, 150, 200, .5)\n    }\n\n    .swal2-file::-moz-placeholder,\n    .swal2-input::-moz-placeholder,\n    .swal2-textarea::-moz-placeholder {\n        color: #ccc\n    }\n\n    .swal2-file:-ms-input-placeholder,\n    .swal2-input:-ms-input-placeholder,\n    .swal2-textarea:-ms-input-placeholder {\n        color: #ccc\n    }\n\n    .swal2-file::placeholder,\n    .swal2-input::placeholder,\n    .swal2-textarea::placeholder {\n        color: #ccc\n    }\n\n    .swal2-range {\n        margin: 1em 2em 3px;\n        background: #fff\n    }\n\n    .swal2-range input {\n        width: 80%\n    }\n\n    .swal2-range output {\n        width: 20%;\n        color: inherit;\n        font-weight: 600;\n        text-align: center\n    }\n\n    .swal2-range input,\n    .swal2-range output {\n        height: 2.625em;\n        padding: 0;\n        font-size: 1.125em;\n        line-height: 2.625em\n    }\n\n    .swal2-input {\n        height: 2.625em;\n        padding: 0 .75em\n    }\n\n    .swal2-file {\n        width: 75%;\n        margin-right: auto;\n        margin-left: auto;\n        background: inherit;\n        font-size: 1.125em\n    }\n\n    .swal2-textarea {\n        height: 6.75em;\n        padding: .75em\n    }\n\n    .swal2-select {\n        min-width: 50%;\n        max-width: 100%;\n        padding: .375em .625em;\n        background: inherit;\n        color: inherit;\n        font-size: 1.125em\n    }\n\n    .swal2-checkbox,\n    .swal2-radio {\n        align-items: center;\n        justify-content: center;\n        background: #fff;\n        color: inherit\n    }\n\n    .swal2-checkbox label,\n    .swal2-radio label {\n        margin: 0 .6em;\n        font-size: 1.125em\n    }\n\n    .swal2-checkbox input,\n    .swal2-radio input {\n        flex-shrink: 0;\n        margin: 0 .4em\n    }\n\n    .swal2-input-label {\n        display: flex;\n        justify-content: center;\n        margin: 1em auto 0\n    }\n\n    .swal2-validation-message {\n        align-items: center;\n        justify-content: center;\n        margin: 1em 0 0;\n        padding: .625em;\n        overflow: hidden;\n        background: #f0f0f0;\n        color: #666;\n        font-size: 1em;\n        font-weight: 300\n    }\n\n    .swal2-validation-message::before {\n        content: \"!\";\n        display: inline-block;\n        width: 1.5em;\n        min-width: 1.5em;\n        height: 1.5em;\n        margin: 0 .625em;\n        border-radius: 50%;\n        background-color: #f27474;\n        color: #fff;\n        font-weight: 600;\n        line-height: 1.5em;\n        text-align: center\n    }\n\n    .swal2-icon {\n        position: relative;\n        box-sizing: content-box;\n        justify-content: center;\n        width: 5em;\n        height: 5em;\n        margin: 2.5em auto .6em;\n        border: .25em solid transparent;\n        border-radius: 50%;\n        border-color: #000;\n        font-family: inherit;\n        line-height: 5em;\n        cursor: default;\n        -webkit-user-select: none;\n        -moz-user-select: none;\n        -ms-user-select: none;\n        user-select: none\n    }\n\n    .swal2-icon .swal2-icon-content {\n        display: flex;\n        align-items: center;\n        font-size: 3.75em\n    }\n\n    .swal2-icon.swal2-error {\n        border-color: #f27474;\n        color: #f27474\n    }\n\n    .swal2-icon.swal2-error .swal2-x-mark {\n        position: relative;\n        flex-grow: 1\n    }\n\n    .swal2-icon.swal2-error [class^=swal2-x-mark-line] {\n        display: block;\n        position: absolute;\n        top: 2.3125em;\n        width: 2.9375em;\n        height: .3125em;\n        border-radius: .125em;\n        background-color: #f27474\n    }\n\n    .swal2-icon.swal2-error [class^=swal2-x-mark-line][class$=left] {\n        left: 1.0625em;\n        transform: rotate(45deg)\n    }\n\n    .swal2-icon.swal2-error [class^=swal2-x-mark-line][class$=right] {\n        right: 1em;\n        transform: rotate(-45deg)\n    }\n\n    .swal2-icon.swal2-error.swal2-icon-show {\n        -webkit-animation: swal2-animate-error-icon .5s;\n        animation: swal2-animate-error-icon .5s\n    }\n\n    .swal2-icon.swal2-error.swal2-icon-show .swal2-x-mark {\n        -webkit-animation: swal2-animate-error-x-mark .5s;\n        animation: swal2-animate-error-x-mark .5s\n    }\n\n    .swal2-icon.swal2-warning {\n        border-color: #facea8;\n        color: #f8bb86\n    }\n\n    .swal2-icon.swal2-warning.swal2-icon-show {\n        -webkit-animation: swal2-animate-error-icon .5s;\n        animation: swal2-animate-error-icon .5s\n    }\n\n    .swal2-icon.swal2-warning.swal2-icon-show .swal2-icon-content {\n        -webkit-animation: swal2-animate-i-mark .5s;\n        animation: swal2-animate-i-mark .5s\n    }\n\n    .swal2-icon.swal2-info {\n        border-color: #9de0f6;\n        color: #3fc3ee\n    }\n\n    .swal2-icon.swal2-info.swal2-icon-show {\n        -webkit-animation: swal2-animate-error-icon .5s;\n        animation: swal2-animate-error-icon .5s\n    }\n\n    .swal2-icon.swal2-info.swal2-icon-show .swal2-icon-content {\n        -webkit-animation: swal2-animate-i-mark .8s;\n        animation: swal2-animate-i-mark .8s\n    }\n\n    .swal2-icon.swal2-question {\n        border-color: #c9dae1;\n        color: #87adbd\n    }\n\n    .swal2-icon.swal2-question.swal2-icon-show {\n        -webkit-animation: swal2-animate-error-icon .5s;\n        animation: swal2-animate-error-icon .5s\n    }\n\n    .swal2-icon.swal2-question.swal2-icon-show .swal2-icon-content {\n        -webkit-animation: swal2-animate-question-mark .8s;\n        animation: swal2-animate-question-mark .8s\n    }\n\n    .swal2-icon.swal2-success {\n        border-color: #a5dc86;\n        color: #a5dc86\n    }\n\n    .swal2-icon.swal2-success [class^=swal2-success-circular-line] {\n        position: absolute;\n        width: 3.75em;\n        height: 7.5em;\n        transform: rotate(45deg);\n        border-radius: 50%\n    }\n\n    .swal2-icon.swal2-success [class^=swal2-success-circular-line][class$=left] {\n        top: -.4375em;\n        left: -2.0635em;\n        transform: rotate(-45deg);\n        transform-origin: 3.75em 3.75em;\n        border-radius: 7.5em 0 0 7.5em\n    }\n\n    .swal2-icon.swal2-success [class^=swal2-success-circular-line][class$=right] {\n        top: -.6875em;\n        left: 1.875em;\n        transform: rotate(-45deg);\n        transform-origin: 0 3.75em;\n        border-radius: 0 7.5em 7.5em 0\n    }\n\n    .swal2-icon.swal2-success .swal2-success-ring {\n        position: absolute;\n        z-index: 2;\n        top: -.25em;\n        left: -.25em;\n        box-sizing: content-box;\n        width: 100%;\n        height: 100%;\n        border: .25em solid rgba(165, 220, 134, .3);\n        border-radius: 50%\n    }\n\n    .swal2-icon.swal2-success .swal2-success-fix {\n        position: absolute;\n        z-index: 1;\n        top: .5em;\n        left: 1.625em;\n        width: .4375em;\n        height: 5.625em;\n        transform: rotate(-45deg)\n    }\n\n    .swal2-icon.swal2-success [class^=swal2-success-line] {\n        display: block;\n        position: absolute;\n        z-index: 2;\n        height: .3125em;\n        border-radius: .125em;\n        background-color: #a5dc86\n    }\n\n    .swal2-icon.swal2-success [class^=swal2-success-line][class$=tip] {\n        top: 2.875em;\n        left: .8125em;\n        width: 1.5625em;\n        transform: rotate(45deg)\n    }\n\n    .swal2-icon.swal2-success [class^=swal2-success-line][class$=long] {\n        top: 2.375em;\n        right: .5em;\n        width: 2.9375em;\n        transform: rotate(-45deg)\n    }\n\n    .swal2-icon.swal2-success.swal2-icon-show .swal2-success-line-tip {\n        -webkit-animation: swal2-animate-success-line-tip .75s;\n        animation: swal2-animate-success-line-tip .75s\n    }\n\n    .swal2-icon.swal2-success.swal2-icon-show .swal2-success-line-long {\n        -webkit-animation: swal2-animate-success-line-long .75s;\n        animation: swal2-animate-success-line-long .75s\n    }\n\n    .swal2-icon.swal2-success.swal2-icon-show .swal2-success-circular-line-right {\n        -webkit-animation: swal2-rotate-success-circular-line 4.25s ease-in;\n        animation: swal2-rotate-success-circular-line 4.25s ease-in\n    }\n\n    .swal2-progress-steps {\n        flex-wrap: wrap;\n        align-items: center;\n        max-width: 100%;\n        margin: 1.25em auto;\n        padding: 0;\n        background: inherit;\n        font-weight: 600\n    }\n\n    .swal2-progress-steps li {\n        display: inline-block;\n        position: relative\n    }\n\n    .swal2-progress-steps .swal2-progress-step {\n        z-index: 20;\n        flex-shrink: 0;\n        width: 2em;\n        height: 2em;\n        border-radius: 2em;\n        background: #2778c4;\n        color: #fff;\n        line-height: 2em;\n        text-align: center\n    }\n\n    .swal2-progress-steps .swal2-progress-step.swal2-active-progress-step {\n        background: #2778c4\n    }\n\n    .swal2-progress-steps .swal2-progress-step.swal2-active-progress-step~.swal2-progress-step {\n        background: #add8e6;\n        color: #fff\n    }\n\n    .swal2-progress-steps .swal2-progress-step.swal2-active-progress-step~.swal2-progress-step-line {\n        background: #add8e6\n    }\n\n    .swal2-progress-steps .swal2-progress-step-line {\n        z-index: 10;\n        flex-shrink: 0;\n        width: 2.5em;\n        height: .4em;\n        margin: 0 -1px;\n        background: #2778c4\n    }\n\n    [class^=swal2] {\n        -webkit-tap-highlight-color: transparent\n    }\n\n    .swal2-show {\n        -webkit-animation: swal2-show .3s;\n        animation: swal2-show .3s\n    }\n\n    .swal2-hide {\n        -webkit-animation: swal2-hide .15s forwards;\n        animation: swal2-hide .15s forwards\n    }\n\n    .swal2-noanimation {\n        transition: none\n    }\n\n    .swal2-scrollbar-measure {\n        position: absolute;\n        top: -9999px;\n        width: 50px;\n        height: 50px;\n        overflow: scroll\n    }\n\n    .swal2-rtl .swal2-close {\n        margin-right: initial;\n        margin-left: 0\n    }\n\n    .swal2-rtl .swal2-timer-progress-bar {\n        right: 0;\n        left: auto\n    }\n\n    @-webkit-keyframes swal2-toast-show {\n        0% {\n            transform: translateY(-.625em) rotateZ(2deg)\n        }\n\n        33% {\n            transform: translateY(0) rotateZ(-2deg)\n        }\n\n        66% {\n            transform: translateY(.3125em) rotateZ(2deg)\n        }\n\n        100% {\n            transform: translateY(0) rotateZ(0)\n        }\n    }\n\n    @keyframes swal2-toast-show {\n        0% {\n            transform: translateY(-.625em) rotateZ(2deg)\n        }\n\n        33% {\n            transform: translateY(0) rotateZ(-2deg)\n        }\n\n        66% {\n            transform: translateY(.3125em) rotateZ(2deg)\n        }\n\n        100% {\n            transform: translateY(0) rotateZ(0)\n        }\n    }\n\n    @-webkit-keyframes swal2-toast-hide {\n        100% {\n            transform: rotateZ(1deg);\n            opacity: 0\n        }\n    }\n\n    @keyframes swal2-toast-hide {\n        100% {\n            transform: rotateZ(1deg);\n            opacity: 0\n        }\n    }\n\n    @-webkit-keyframes swal2-toast-animate-success-line-tip {\n        0% {\n            top: .5625em;\n            left: .0625em;\n            width: 0\n        }\n\n        54% {\n            top: .125em;\n            left: .125em;\n            width: 0\n        }\n\n        70% {\n            top: .625em;\n            left: -.25em;\n            width: 1.625em\n        }\n\n        84% {\n            top: 1.0625em;\n            left: .75em;\n            width: .5em\n        }\n\n        100% {\n            top: 1.125em;\n            left: .1875em;\n            width: .75em\n        }\n    }\n\n    @keyframes swal2-toast-animate-success-line-tip {\n        0% {\n            top: .5625em;\n            left: .0625em;\n            width: 0\n        }\n\n        54% {\n            top: .125em;\n            left: .125em;\n            width: 0\n        }\n\n        70% {\n            top: .625em;\n            left: -.25em;\n            width: 1.625em\n        }\n\n        84% {\n            top: 1.0625em;\n            left: .75em;\n            width: .5em\n        }\n\n        100% {\n            top: 1.125em;\n            left: .1875em;\n            width: .75em\n        }\n    }\n\n    @-webkit-keyframes swal2-toast-animate-success-line-long {\n        0% {\n            top: 1.625em;\n            right: 1.375em;\n            width: 0\n        }\n\n        65% {\n            top: 1.25em;\n            right: .9375em;\n            width: 0\n        }\n\n        84% {\n            top: .9375em;\n            right: 0;\n            width: 1.125em\n        }\n\n        100% {\n            top: .9375em;\n            right: .1875em;\n            width: 1.375em\n        }\n    }\n\n    @keyframes swal2-toast-animate-success-line-long {\n        0% {\n            top: 1.625em;\n            right: 1.375em;\n            width: 0\n        }\n\n        65% {\n            top: 1.25em;\n            right: .9375em;\n            width: 0\n        }\n\n        84% {\n            top: .9375em;\n            right: 0;\n            width: 1.125em\n        }\n\n        100% {\n            top: .9375em;\n            right: .1875em;\n            width: 1.375em\n        }\n    }\n\n    @-webkit-keyframes swal2-show {\n        0% {\n            transform: scale(.7)\n        }\n\n        45% {\n            transform: scale(1.05)\n        }\n\n        80% {\n            transform: scale(.95)\n        }\n\n        100% {\n            transform: scale(1)\n        }\n    }\n\n    @keyframes swal2-show {\n        0% {\n            transform: scale(.7)\n        }\n\n        45% {\n            transform: scale(1.05)\n        }\n\n        80% {\n            transform: scale(.95)\n        }\n\n        100% {\n            transform: scale(1)\n        }\n    }\n\n    @-webkit-keyframes swal2-hide {\n        0% {\n            transform: scale(1);\n            opacity: 1\n        }\n\n        100% {\n            transform: scale(.5);\n            opacity: 0\n        }\n    }\n\n    @keyframes swal2-hide {\n        0% {\n            transform: scale(1);\n            opacity: 1\n        }\n\n        100% {\n            transform: scale(.5);\n            opacity: 0\n        }\n    }\n\n    @-webkit-keyframes swal2-animate-success-line-tip {\n        0% {\n            top: 1.1875em;\n            left: .0625em;\n            width: 0\n        }\n\n        54% {\n            top: 1.0625em;\n            left: .125em;\n            width: 0\n        }\n\n        70% {\n            top: 2.1875em;\n            left: -.375em;\n            width: 3.125em\n        }\n\n        84% {\n            top: 3em;\n            left: 1.3125em;\n            width: 1.0625em\n        }\n\n        100% {\n            top: 2.8125em;\n            left: .8125em;\n            width: 1.5625em\n        }\n    }\n\n    @keyframes swal2-animate-success-line-tip {\n        0% {\n            top: 1.1875em;\n            left: .0625em;\n            width: 0\n        }\n\n        54% {\n            top: 1.0625em;\n            left: .125em;\n            width: 0\n        }\n\n        70% {\n            top: 2.1875em;\n            left: -.375em;\n            width: 3.125em\n        }\n\n        84% {\n            top: 3em;\n            left: 1.3125em;\n            width: 1.0625em\n        }\n\n        100% {\n            top: 2.8125em;\n            left: .8125em;\n            width: 1.5625em\n        }\n    }\n\n    @-webkit-keyframes swal2-animate-success-line-long {\n        0% {\n            top: 3.375em;\n            right: 2.875em;\n            width: 0\n        }\n\n        65% {\n            top: 3.375em;\n            right: 2.875em;\n            width: 0\n        }\n\n        84% {\n            top: 2.1875em;\n            right: 0;\n            width: 3.4375em\n        }\n\n        100% {\n            top: 2.375em;\n            right: .5em;\n            width: 2.9375em\n        }\n    }\n\n    @keyframes swal2-animate-success-line-long {\n        0% {\n            top: 3.375em;\n            right: 2.875em;\n            width: 0\n        }\n\n        65% {\n            top: 3.375em;\n            right: 2.875em;\n            width: 0\n        }\n\n        84% {\n            top: 2.1875em;\n            right: 0;\n            width: 3.4375em\n        }\n\n        100% {\n            top: 2.375em;\n            right: .5em;\n            width: 2.9375em\n        }\n    }\n\n    @-webkit-keyframes swal2-rotate-success-circular-line {\n        0% {\n            transform: rotate(-45deg)\n        }\n\n        5% {\n            transform: rotate(-45deg)\n        }\n\n        12% {\n            transform: rotate(-405deg)\n        }\n\n        100% {\n            transform: rotate(-405deg)\n        }\n    }\n\n    @keyframes swal2-rotate-success-circular-line {\n        0% {\n            transform: rotate(-45deg)\n        }\n\n        5% {\n            transform: rotate(-45deg)\n        }\n\n        12% {\n            transform: rotate(-405deg)\n        }\n\n        100% {\n            transform: rotate(-405deg)\n        }\n    }\n\n    @-webkit-keyframes swal2-animate-error-x-mark {\n        0% {\n            margin-top: 1.625em;\n            transform: scale(.4);\n            opacity: 0\n        }\n\n        50% {\n            margin-top: 1.625em;\n            transform: scale(.4);\n            opacity: 0\n        }\n\n        80% {\n            margin-top: -.375em;\n            transform: scale(1.15)\n        }\n\n        100% {\n            margin-top: 0;\n            transform: scale(1);\n            opacity: 1\n        }\n    }\n\n    @keyframes swal2-animate-error-x-mark {\n        0% {\n            margin-top: 1.625em;\n            transform: scale(.4);\n            opacity: 0\n        }\n\n        50% {\n            margin-top: 1.625em;\n            transform: scale(.4);\n            opacity: 0\n        }\n\n        80% {\n            margin-top: -.375em;\n            transform: scale(1.15)\n        }\n\n        100% {\n            margin-top: 0;\n            transform: scale(1);\n            opacity: 1\n        }\n    }\n\n    @-webkit-keyframes swal2-animate-error-icon {\n        0% {\n            transform: rotateX(100deg);\n            opacity: 0\n        }\n\n        100% {\n            transform: rotateX(0);\n            opacity: 1\n        }\n    }\n\n    @keyframes swal2-animate-error-icon {\n        0% {\n            transform: rotateX(100deg);\n            opacity: 0\n        }\n\n        100% {\n            transform: rotateX(0);\n            opacity: 1\n        }\n    }\n\n    @-webkit-keyframes swal2-rotate-loading {\n        0% {\n            transform: rotate(0)\n        }\n\n        100% {\n            transform: rotate(360deg)\n        }\n    }\n\n    @keyframes swal2-rotate-loading {\n        0% {\n            transform: rotate(0)\n        }\n\n        100% {\n            transform: rotate(360deg)\n        }\n    }\n\n    @-webkit-keyframes swal2-animate-question-mark {\n        0% {\n            transform: rotateY(-360deg)\n        }\n\n        100% {\n            transform: rotateY(0)\n        }\n    }\n\n    @keyframes swal2-animate-question-mark {\n        0% {\n            transform: rotateY(-360deg)\n        }\n\n        100% {\n            transform: rotateY(0)\n        }\n    }\n\n    @-webkit-keyframes swal2-animate-i-mark {\n        0% {\n            transform: rotateZ(45deg);\n            opacity: 0\n        }\n\n        25% {\n            transform: rotateZ(-25deg);\n            opacity: .4\n        }\n\n        50% {\n            transform: rotateZ(15deg);\n            opacity: .8\n        }\n\n        75% {\n            transform: rotateZ(-5deg);\n            opacity: 1\n        }\n\n        100% {\n            transform: rotateX(0);\n            opacity: 1\n        }\n    }\n\n    @keyframes swal2-animate-i-mark {\n        0% {\n            transform: rotateZ(45deg);\n            opacity: 0\n        }\n\n        25% {\n            transform: rotateZ(-25deg);\n            opacity: .4\n        }\n\n        50% {\n            transform: rotateZ(15deg);\n            opacity: .8\n        }\n\n        75% {\n            transform: rotateZ(-5deg);\n            opacity: 1\n        }\n\n        100% {\n            transform: rotateX(0);\n            opacity: 1\n        }\n    }\n\n    body.swal2-shown:not(.swal2-no-backdrop):not(.swal2-toast-shown) {\n        overflow: hidden\n    }\n\n    body.swal2-height-auto {\n        height: auto !important\n    }\n\n    body.swal2-no-backdrop .swal2-container {\n        background-color: transparent !important;\n        pointer-events: none\n    }\n\n    body.swal2-no-backdrop .swal2-container .swal2-popup {\n        pointer-events: all\n    }\n\n    body.swal2-no-backdrop .swal2-container .swal2-modal {\n        box-shadow: 0 0 10px rgba(0, 0, 0, .4)\n    }\n\n    @media print {\n        body.swal2-shown:not(.swal2-no-backdrop):not(.swal2-toast-shown) {\n            overflow-y: scroll !important\n        }\n\n        body.swal2-shown:not(.swal2-no-backdrop):not(.swal2-toast-shown)>[aria-hidden=true] {\n            display: none\n        }\n\n        body.swal2-shown:not(.swal2-no-backdrop):not(.swal2-toast-shown) .swal2-container {\n            position: static !important\n        }\n    }\n\n    body.swal2-toast-shown .swal2-container {\n        box-sizing: border-box;\n        width: 360px;\n        max-width: 100%;\n        background-color: transparent;\n        pointer-events: none\n    }\n\n    body.swal2-toast-shown .swal2-container.swal2-top {\n        top: 0;\n        right: auto;\n        bottom: auto;\n        left: 50%;\n        transform: translateX(-50%)\n    }\n\n    body.swal2-toast-shown .swal2-container.swal2-top-end,\n    body.swal2-toast-shown .swal2-container.swal2-top-right {\n        top: 0;\n        right: 0;\n        bottom: auto;\n        left: auto\n    }\n\n    body.swal2-toast-shown .swal2-container.swal2-top-left,\n    body.swal2-toast-shown .swal2-container.swal2-top-start {\n        top: 0;\n        right: auto;\n        bottom: auto;\n        left: 0\n    }\n\n    body.swal2-toast-shown .swal2-container.swal2-center-left,\n    body.swal2-toast-shown .swal2-container.swal2-center-start {\n        top: 50%;\n        right: auto;\n        bottom: auto;\n        left: 0;\n        transform: translateY(-50%)\n    }\n\n    body.swal2-toast-shown .swal2-container.swal2-center {\n        top: 50%;\n        right: auto;\n        bottom: auto;\n        left: 50%;\n        transform: translate(-50%, -50%)\n    }\n\n    body.swal2-toast-shown .swal2-container.swal2-center-end,\n    body.swal2-toast-shown .swal2-container.swal2-center-right {\n        top: 50%;\n        right: 0;\n        bottom: auto;\n        left: auto;\n        transform: translateY(-50%)\n    }\n\n    body.swal2-toast-shown .swal2-container.swal2-bottom-left,\n    body.swal2-toast-shown .swal2-container.swal2-bottom-start {\n        top: auto;\n        right: auto;\n        bottom: 0;\n        left: 0\n    }\n\n    body.swal2-toast-shown .swal2-container.swal2-bottom {\n        top: auto;\n        right: auto;\n        bottom: 0;\n        left: 50%;\n        transform: translateX(-50%)\n    }\n\n    body.swal2-toast-shown .swal2-container.swal2-bottom-end,\n    body.swal2-toast-shown .swal2-container.swal2-bottom-right {\n        top: auto;\n        right: 0;\n        bottom: 0;\n        left: auto\n    }\n</style>\n"  # HTML Header
  n1 = Concatenate Strings(w4, "\n", w2) -> (w1:string)
  n2 = case shown="No Error" "Error In" {
    selector: "Error In" -> [w17 w19]
    tunnel: [w12 w19] -> w8
    tunnel: [w13 w18] -> w6
    tunnel: "reference in" -> [w16 w18]
    tunnel: [w11 _] -> w5
    tunnel: w1 -> [w10 _]
    frame No Error {
      n3 = call "LcWebView_GetAttributes.vi"("reference in"=w16, "error in (no error)"=w17) -> ("reference out"=w14:refnum<class "LcWebView.lvclass">, "error out"=w15:errorcluster)  [unwired: 14 in, 2 out]
      n4 = call-dynamic "NavigateToString.vi"("reference in"=w14, "HTML Content"=w10, "Error In"=w15) -> ("reference out"=w13:refnum<class "LcWebView.lvclass">, "Loaded"=w11:bool, "Error Out"=w12:errorcluster)  [unwired: 14 in]
    }
    frame Error {
    }
  }
  "Error Out" <- w8
  "reference out" <- w6
  "Loaded" <- w5
